vi "DB Message Loop.vi"(8 "error in (no error)":errorcluster, 11 "Message Queues":T1) -> (0 "error out":errorcluster)   [LabVIEW 2026, in "Database.lvlib"]
uses:
  Database.lvlib
  support/Architecture/Message Queue/All Message Queues.ctl
  support/Architecture/Message Queue/Message Cluster.ctl
  <vilib>/addons/database/Connection.llb/Conn ObjectReference.ctl
  controls/Loop Memory/DB Session Data.ctl
  controls/UI/Folder Name.ctl
  controls/Messaging Payloads/DB Query Request Payload.ctl
  controls/UI/UI List Type.ctl
  controls/UI/Data Entity.ctl
  controls/UI/Measurement Role Selection.ctl
  controls/Messaging Payloads/Fetch SensorID Payload.ctl
  controls/Messaging Payloads/MSG FetchSensorID Payload.ctl
  controls/Messaging Payloads/Fetch Config Payload.ctl
  controls/Messaging Payloads/MSG FetchConfiguration Payload.ctl
  Acquisition/Instrument Specifications Cluster Configuration.ctl
  controls/UI/Measurement Role.ctl
  controls/Messaging Payloads/Sensor FetchResponse.ctl
  controls/Messaging Payloads/Sensor CoreData Cluster.ctl
  controls/UI/Units Enum.ctl
  controls/UI/Signal Enum.ctl
  controls/UI/Settings Cluster.ctl
  controls/UI/Acq Settings.ctl
  Acquisition/Instrument Specifications Configuration.ctl
  controls/UI/Config Settings.ctl
  Processing/Processing Settings.ctl
  controls/Messaging Payloads/Sensor CoreData.ctl
  Processing/Test Parameters.ctl
  Processing/Test Parameters Cluster.ctl
  controls/UI/Test Sequence Context.ctl
  controls/UI/Direction.ctl
  controls/UI/Session Identfiers.ctl
  controls/UI/Test Sequence Settings.ctl
  controls/UI/Test Sequence State.ctl
  controls/UI/Test Sequence Enum.ctl
  controls/Controller/Stimulus Settings.ctl
  controls/Controller/Stimulus Outputs.ctl
  controls/Controller/Stimulus Output.ctl
  controls/Controller/Controller Core Data.ctl
  controls/Controller/Stimulus Output Configuration.ctl
  controls/Controller/Stimulus Role.ctl
  controls/Messaging Payloads/TestRuns Table Insert.ctl
  controls/Messaging Payloads/DB TestRunChannel Record.ctl
  controls/Messaging Payloads/Sensor InsertRequest.ctl
  controls/Diagnostics/Error Cluster.ctl
  controls/Messaging Payloads/Sensor Table Insert.ctl
  controls/Diagnostics/Error Payload.ctl
  controls/Messaging Payloads/Channel InsertRequest.ctl
  controls/Messaging Payloads/Channel CoreData Cluster.ctl
  controls/Messaging Payloads/Operator InsertRequest.ctl
  controls/Messaging Payloads/Processed Calibration Points.ctl
  controls/Messaging Payloads/Processed Calibration Point.ctl
  Processing/Test Status.ctl
  controls/Messaging Payloads/Calibration Point Table Insert.ctl
  controls/Diagnostics/Error_Payload.ctl
  <vilib>/addons/database/Connection.llb/DB Tools Open Connec (String).vi
  <vilib>/addons/database/Connection.llb/Conn Execute.vi
  <vilib>/addons/database/Recordset.llb/Rec Destroy - Connection.vi
  <vilib>/addons/database/Recordset.llb/Rec Fetch Integer Data (R).vi
  <vilib>/Utility/error.llb/Error Cluster From Error Code.vi
  <vilib>/ErrorRing/Error Ring.xnode
  <vilib>/addons/database/NI_Database_API.lvlib
  support/Architecture/Message Queue/Message Queue.lvlib
  Acquisition/Acquisition.lvlib
  Settings/Settings.lvlib
  Processing/Processing_Engine.lvlib
  Analysis/Analysis.lvlib
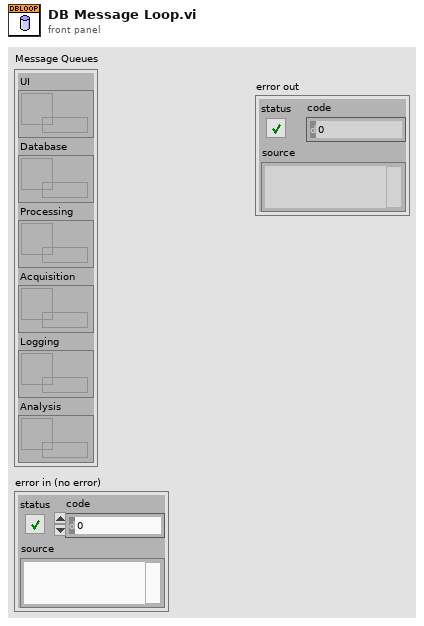
[diagram p1: front panel]
types:
  T1 = typedef "Message Queue.lvlib/All Message Queues.ctl" = cluster{"UI":refnum<queue>, "Database":refnum<queue>, "Processing":refnum<queue>, "Acquisition":refnum<queue>, "Logging":refnum<queue>, "Analysis":refnum<queue>}
  T2 = typedef "Folder Name.ctl" = enum16{"Data", "TDMS"}
  T3 = typedef "Settings.lvlib/Measurement Role Selection.ctl" = enum16{"Controller", "Reference", "UUT", "All"}
  T4 = typedef "UI List Type.ctl" = enum16{"Model Numbers", "Serial Numbers", "Operators", "Calibration Points", "Start Run Times"}
  T5 = typedef "Settings.lvlib/Measurement Role.ctl" = enum16{"Reference", "UUT"}
  T6 = typedef "DB Session Data.ctl" = cluster{"SensorID":i32[], "OperatorID":i32, "TestRunID":i32, "ChannelRecordIDs":i32[], "CalibrationSessionID":i32}
  T7 = typedef "NI_Database_API.lvlib/Conn ObjectReference.ctl" = refnum<k1>
  T8 = typedef "NI_Database_API.lvlib/Rec ObjectReference.ctl" = refnum<k1>
  T9 = typedef "DB Query Request Payload.ctl" = cluster{"1D Notifier":refnum<notifier>, "UI List Type":T4, "UI Device Type":T10, "Identifier":i32, "2D Notifier":refnum<notifier>, "Measurement Role Selection":T3}
  T10 = typedef "Settings.lvlib/Data Entity.ctl" = enum16{"Measurement", "Controller", " Test Configuration"}
  T11 = typedef "Database.lvlib/MSG FetchSensorID Payload.ctl" = cluster{"SensorID":i32, "Serial Number":string, "Model Number":string}
  T12 = typedef "Database.lvlib/Fetch SensorID Payload.ctl" = cluster{"Notifier":refnum<notifier>, "MSG FetchSensorID Payload":T11}
  T13 = typedef "MSG FetchConfiguration Payload.ctl" = cluster{"Serial Numbers":string[], "Hardware Settings Cluster":T14}
  T14 = typedef "Acquisition.lvlib/Instrument Specifications Cluster Configuration.ctl" = cluster{"Sensor ID *":i32, "Target Sample Rate (Hz) *":dbl, "Steady-State Duration (s) *":i32, "Allowed Tolerance (%) FS *":dbl, "Max Settling Timeout (s) *":i32, "Physical Channel":string, "Measurement Role":T5}
  T15 = typedef "Fetch Config Payload.ctl" = cluster{"Model Number":string, "Notifier":refnum<notifier>, "UI Device Type":T10}
  T16 = typedef "Sensor FetchResponse.ctl" = cluster{"Notifier":refnum<notifier>, "Sensor ID":i32}
  T17 = typedef "Settings.lvlib/Sensor CoreData Cluster.ctl" = cluster{"SerialNumber":string, "ModelNumber":string, "Min":dbl, "Max":dbl, "Units":T18, "Output Signal":T19, "SensorID":i32}
  T18 = typedef "Units Enum.ctl" = enum16{"PSI", "Deg C", "kPa", "GPM"}
  T19 = typedef "Signal Enum.ctl" = enum16{"4-20mA", "0-10V", "Thermocouple Type K"}
  T20 = typedef "Settings Cluster.ctl" = cluster{"Acq Settings":T21, "Processing Settings":T24, "Session Identifiers":T30, "Test Sequence Settings":T31, "Stimulus Settings":T34}
  T21 = typedef "Acq Settings.ctl" = cluster{"Instrument Specifications":T22, "Config Settings":T23}
  T22 = typedef "Acquisition.lvlib/Instrument Specifications Configuration.ctl" = T14[]
  T23 = typedef "Config Settings.ctl" = cluster{"Simulated Sensor Injection":dbl, "Base Device Name":string, "Simulation Mode":string}
  T24 = typedef "Processing_Engine.lvlib/Processing Settings.ctl" = cluster{"Sensor CoreData":T25, "Test Parameters":T26, "Measurement Roles":T5[], "Test Sequence Context":T28}
  T25 = typedef "Sensor CoreData.ctl" = T17[]
  T26 = typedef "Processing_Engine.lvlib/Test Parameters.ctl" = T27[]
  T27 = typedef "Settings.lvlib/Test Parameters Cluster.ctl" = cluster{"Steady-State Duration (s)":i32, "Allowed Tolerance (%) FS":dbl, "Max Settling Timeout (s)":i32}
  T28 = typedef "Settings.lvlib/Test Sequence Context.ctl" = cluster{"Direction":T29, "Cycle Number":i32, "Setpoint":dbl}
  T29 = typedef "Settings.lvlib/Direction.ctl" = enum16{"Acsending", "Descending"}
  T30 = typedef "Session Identfiers.ctl" = cluster{"SerialNumber":string[], "OperatorName":string}
  T31 = typedef "Test Sequence Settings.ctl" = cluster{"Test Sequence State":T32}
  T32 = typedef "Settings.lvlib/Test Sequence State.ctl" = cluster{"Test Sequence Enum":T33, "Point Index":i32, "Current Target":dbl, "Previous Target":dbl, "Simulation?":bool, "Direction":T29, "Transition Active?":bool, "Cycle Number":i32}
  T33 = typedef "Test Sequence Enum.ctl" = enum16{"Idle", "Start Point", "Point Complete", "Test Complete", "Abort Test", "Reset"}
  T34 = typedef "Settings.lvlib/Stimulus Settings.ctl" = cluster{"Stimulus Outputs":T35}
  T35 = typedef "Settings.lvlib/Stimulus Outputs.ctl" = T36[]
  T36 = typedef "Settings.lvlib/Stimulus Output.ctl" = cluster{"Controller Core Data":T37, "Stimulus Output Configuration":T38}
  T37 = typedef "Settings.lvlib/Controller Core Data.ctl" = cluster{"Min":dbl, "Max":dbl, "Units":T18, "Input Signal Type":T19, "Input Signal Min":dbl, "Input Signal Max":dbl}
  T38 = typedef "Settings.lvlib/Stimulus Output Configuration.ctl" = cluster{"DAQmx AO Physical Channel":tag, "Role":T39, "Model Numbers":string, "Serial Numbers":string, "Row":i32}
  T39 = typedef "Stimulus Role.ctl" = enum16{"Pressure Controller", "Temperature Controller"}
  T40 = typedef "TestRuns Table Insert.ctl" = cluster{"RunStartTime":string, "OperatorID":i32, "TestResult":string, "CalibrationSessionID":i32}
  T41 = typedef "Database.lvlib/DB TestRunChannel Record.ctl" = cluster{"TestRunID":i32, "SensorID":i32, "HardwareRow":i32, "PhysicalChannel":string, "FinalStatus":string, "MeasurementRole":string}
  T42 = typedef "Settings.lvlib/Sensor Table Insert.ctl" = cluster{"SerialNumber":string, "ModelNumber":string, "Min":dbl, "Max":dbl, "Units":T18, "Output Signal":T19}
  T43 = typedef "Sensor InsertRequest.ctl" = cluster{"Notifier":refnum<notifier>, "Sensor CoreData":T17}
  T44 = typedef "Error Cluster.ctl" = errorcluster
  T45 = typedef "Error Payload.ctl" = cluster{"Error Cluster":T44, "Message":string}
  T46 = typedef "Settings.lvlib/Channel CoreData Cluster.ctl" = cluster{"RunID":i32, "SensorID":i32, "HardwareRow":i32, "PhysicalChannel":string}
  T47 = typedef "Settings.lvlib/Channel InsertRequest.ctl" = cluster{"Notifier":refnum<notifier>, "Channel CoreData":T46}
  T48 = typedef "Operator InsertRequest.ctl" = cluster{"Notifier":refnum<notifier>, "OperatorName":string, "BadgeNumber":string, "IsActive":i32}
  T49 = typedef "Processed Calibration Points.ctl" = T50[]
  T50 = typedef "Processed Calibration Point.ctl" = cluster{"Reference Value":dbl, "Measured Value":dbl, "AccuracyPercentFS":dbl, "Pass/Fail":bool, "Setpoint":dbl, "Cycle Number":i32, "Direction":T29, "Test Status":T51}
  T51 = typedef "Analysis.lvlib/Test Status.ctl" = enum16{"Overall Pass", "Overall Fail", "Test Running"}
  T52 = typedef "Calibration Point Table Insert.ctl" = cluster{"TestRunID":i32, "ChannelRecordID":i32, "Setpoint":dbl, "MeasuredValue":dbl, "AccuracyPercentFS":dbl, "PassFail":bool, "ReferenceValue":dbl, "Cycle Number":i32, "Direction":string, "SensorID":i32}
  T53 = typedef "Error_Payload.ctl" = cluster{"status":bool, "error_code":i32, "description":string, "source_loop":string}
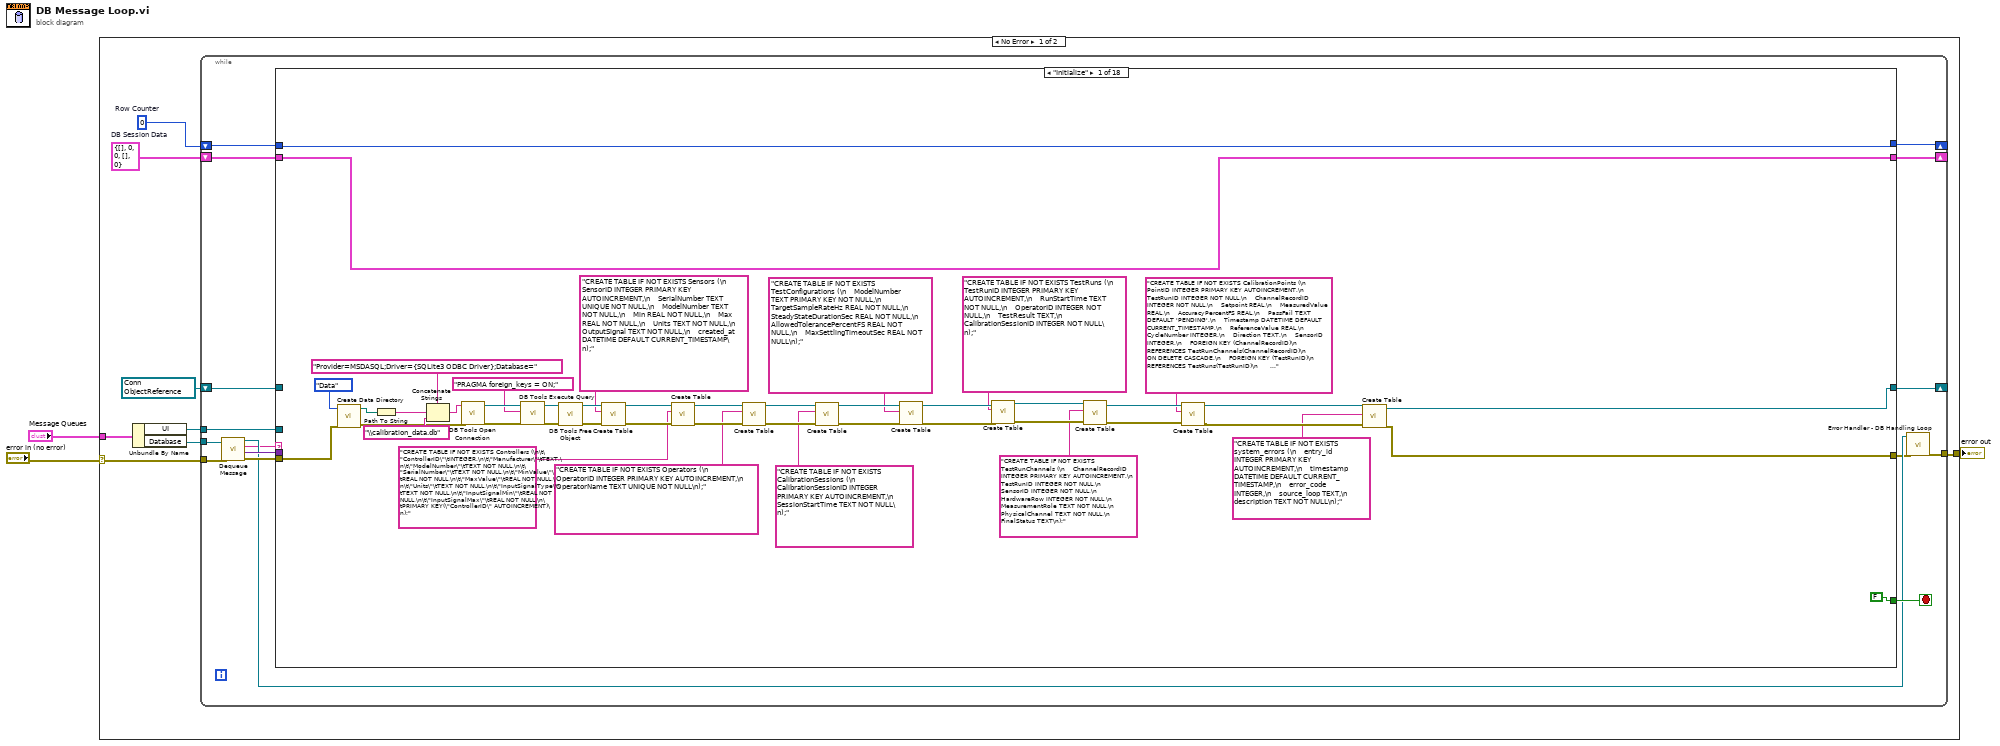
[diagram p0: block diagram]
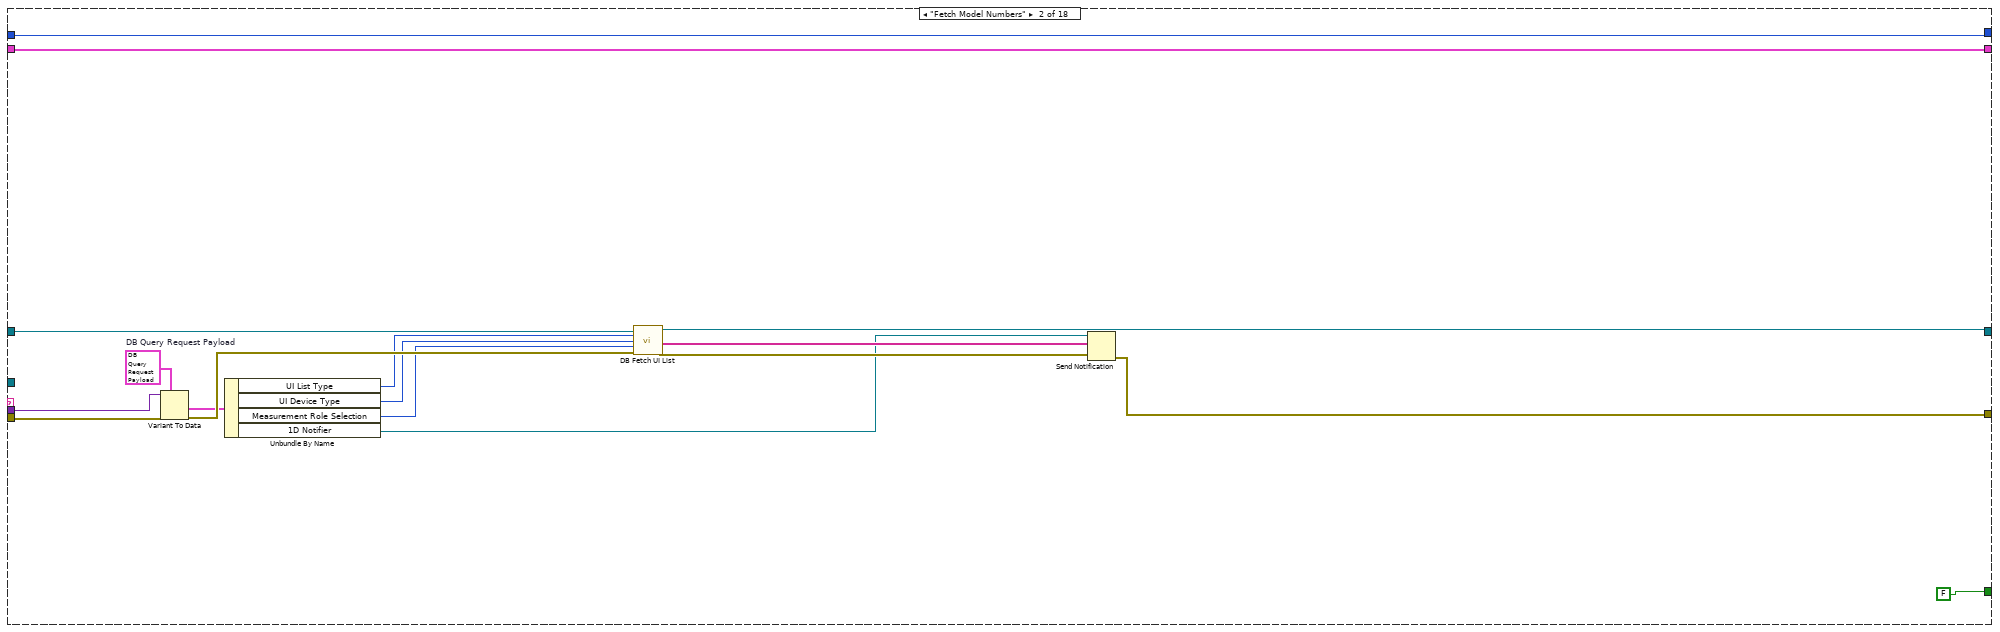
[diagram p2: hidden frame]
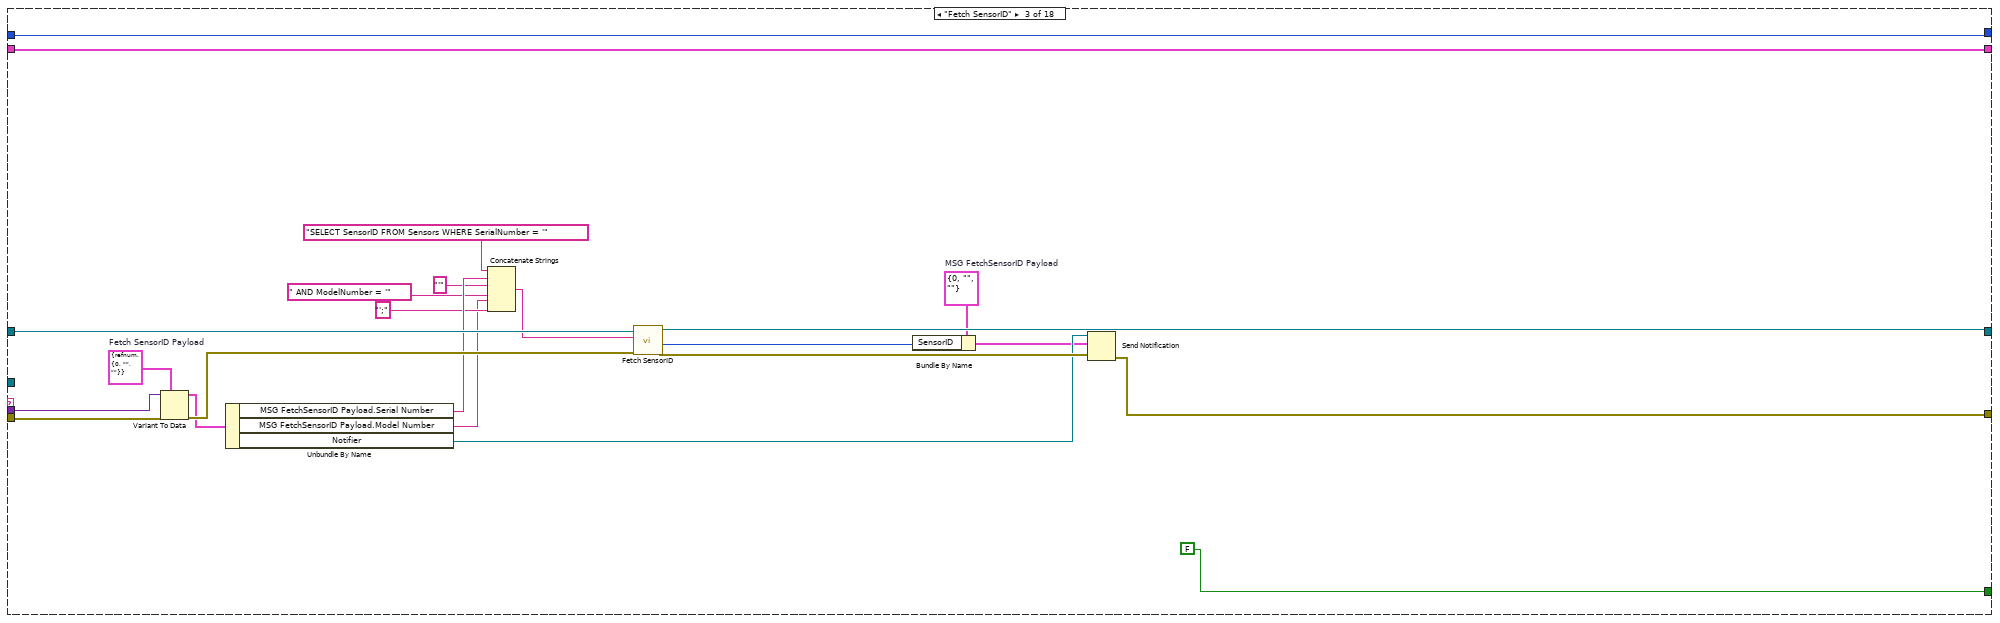
[diagram p3: hidden frame]
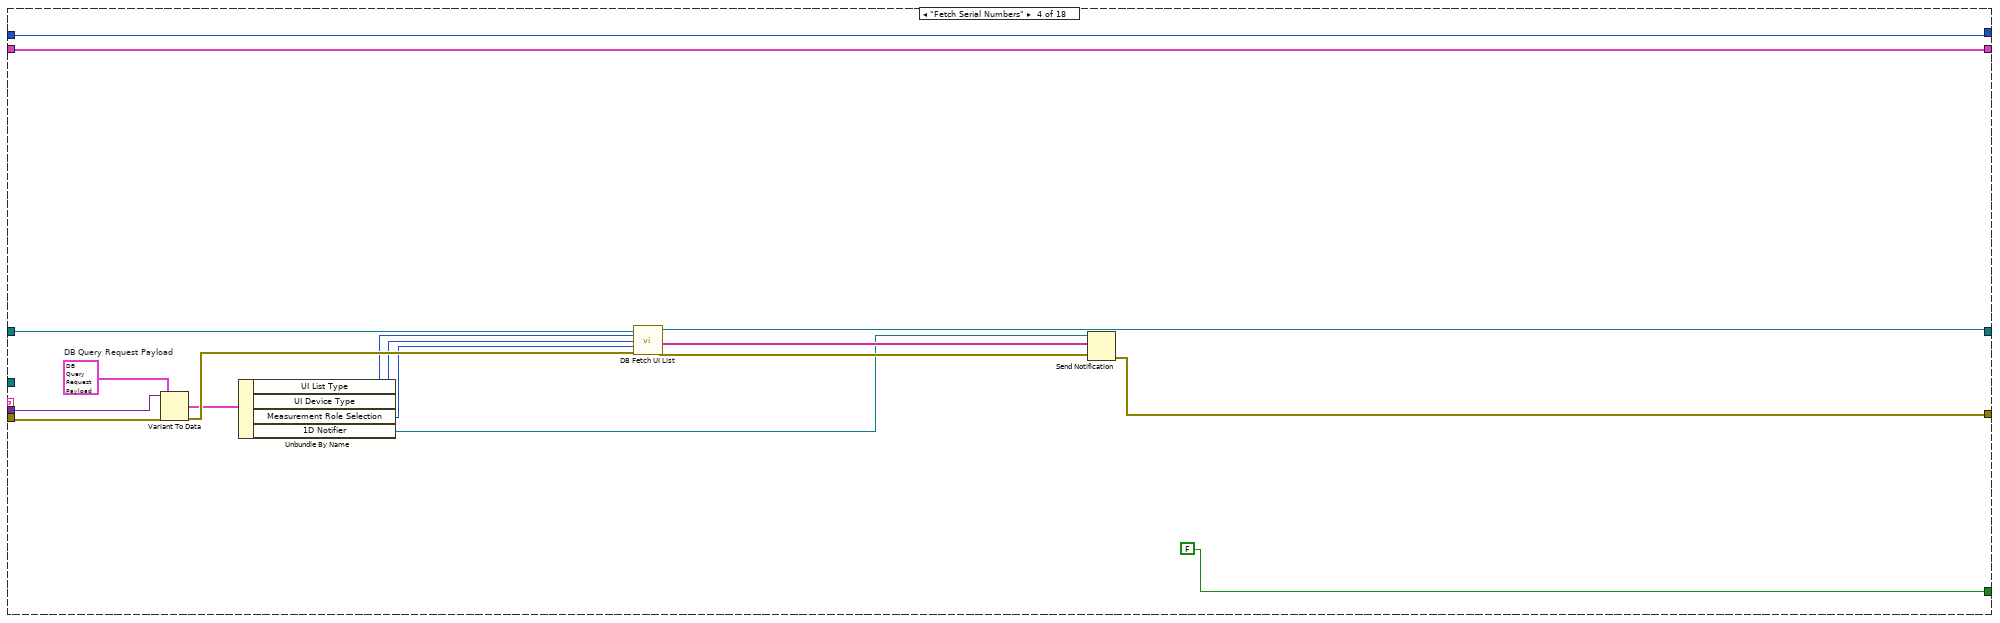
[diagram p4: hidden frame]
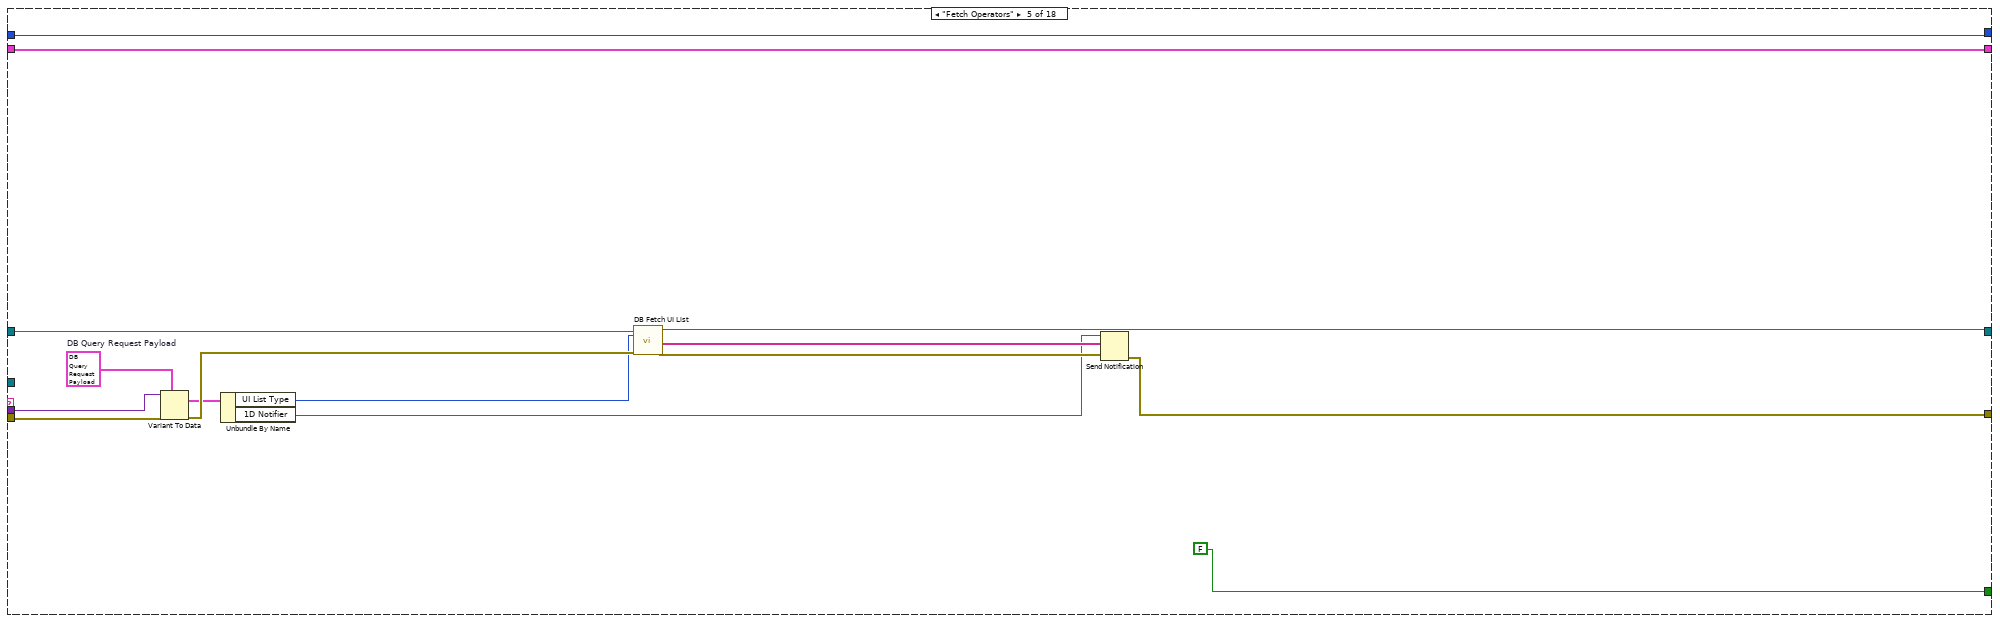
[diagram p5: hidden frame]
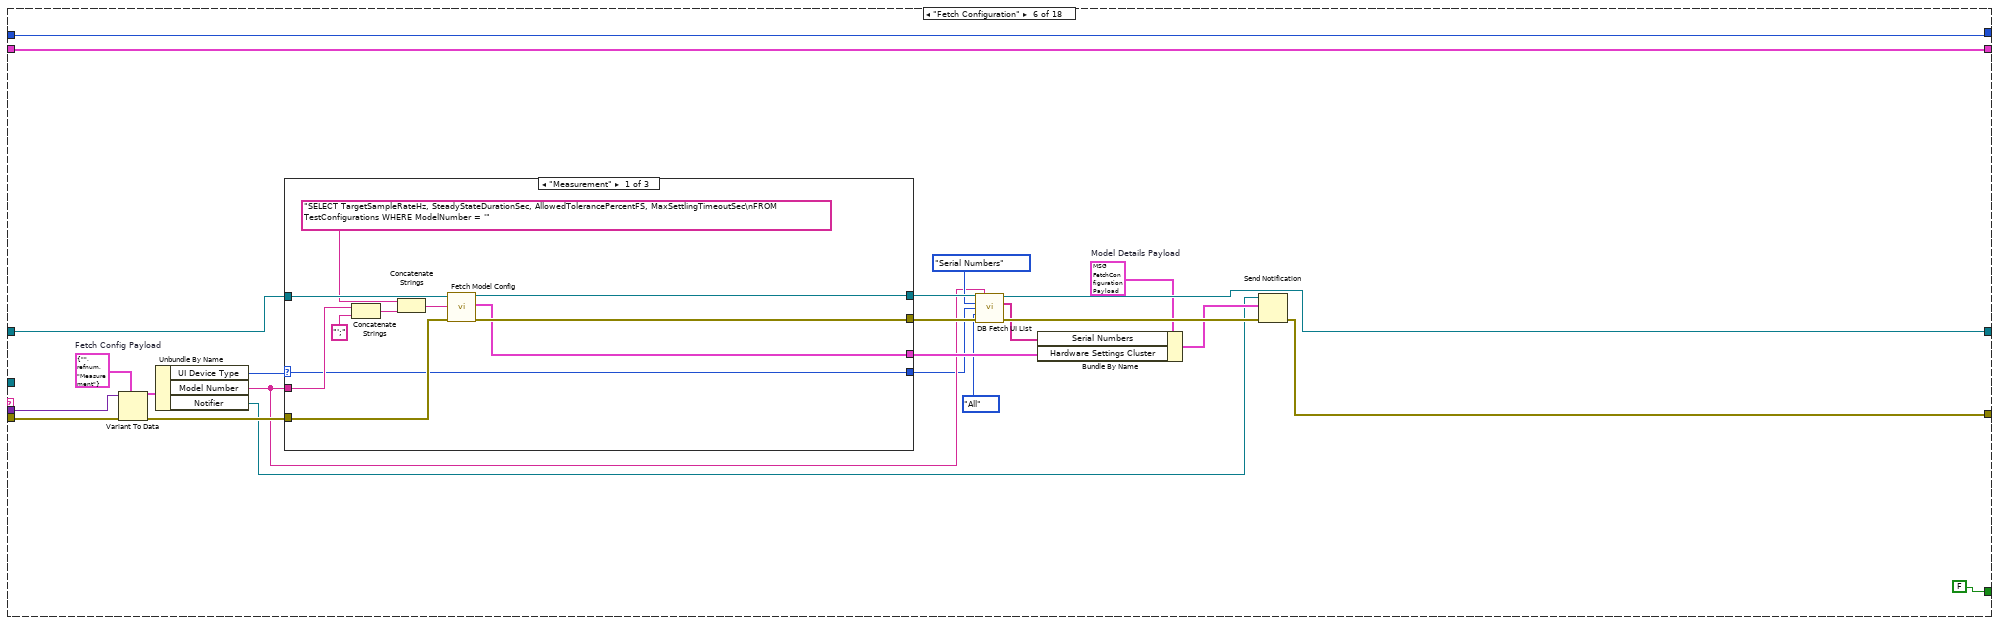
[diagram p6: hidden frame]
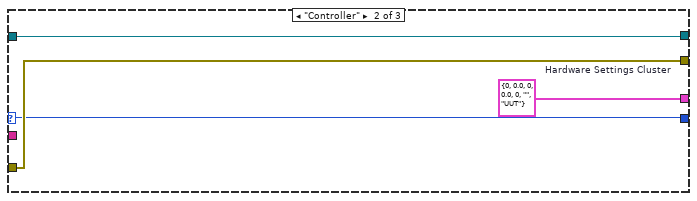
[diagram p7: hidden frame]
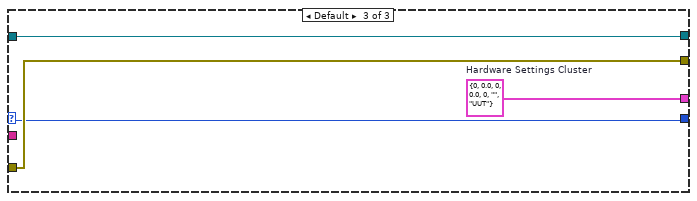
[diagram p8: hidden frame]
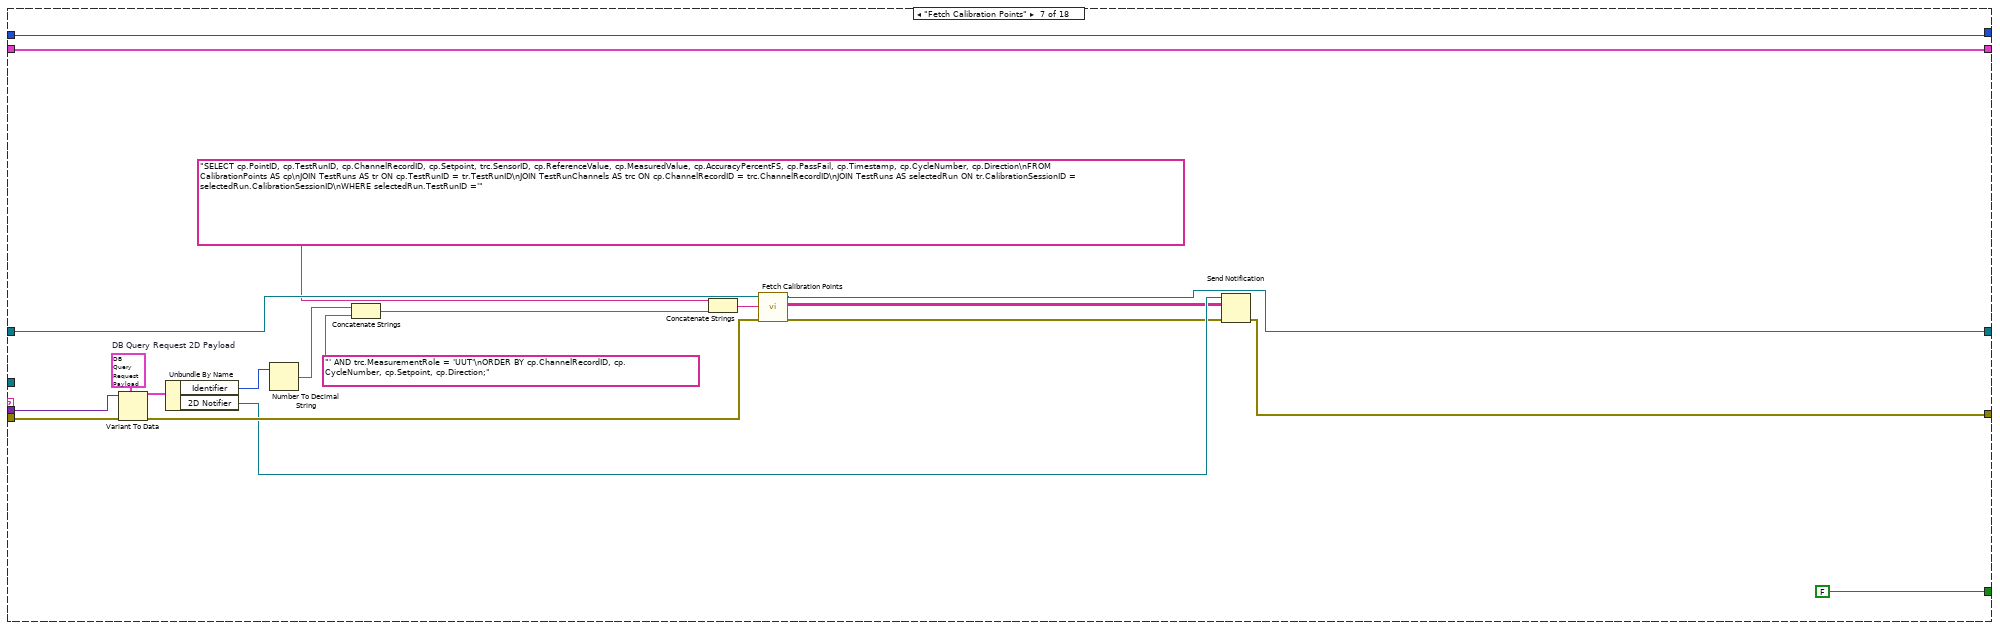
[diagram p9: hidden frame]
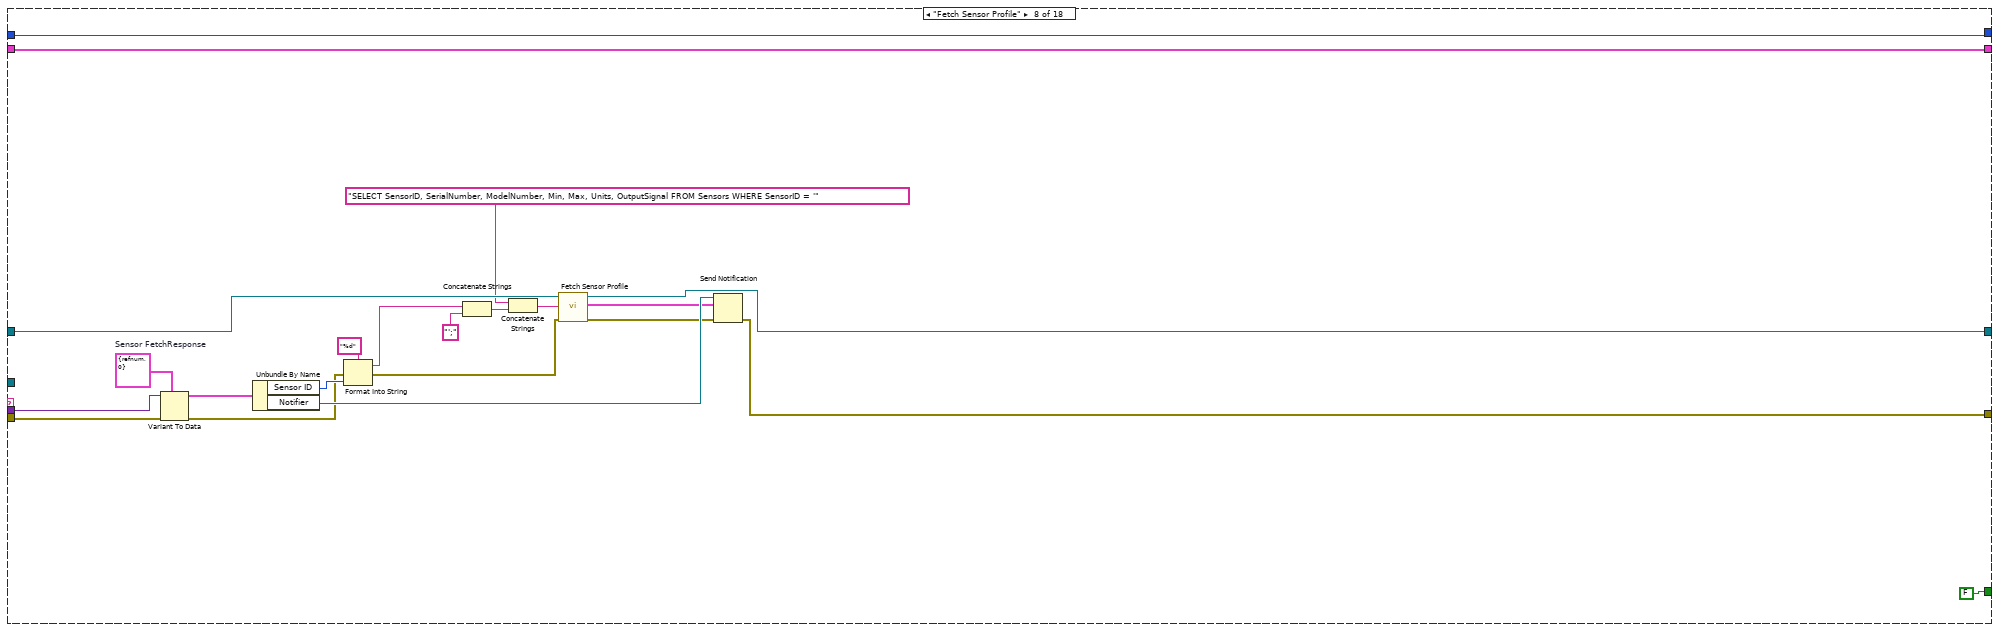
[diagram p10: hidden frame]
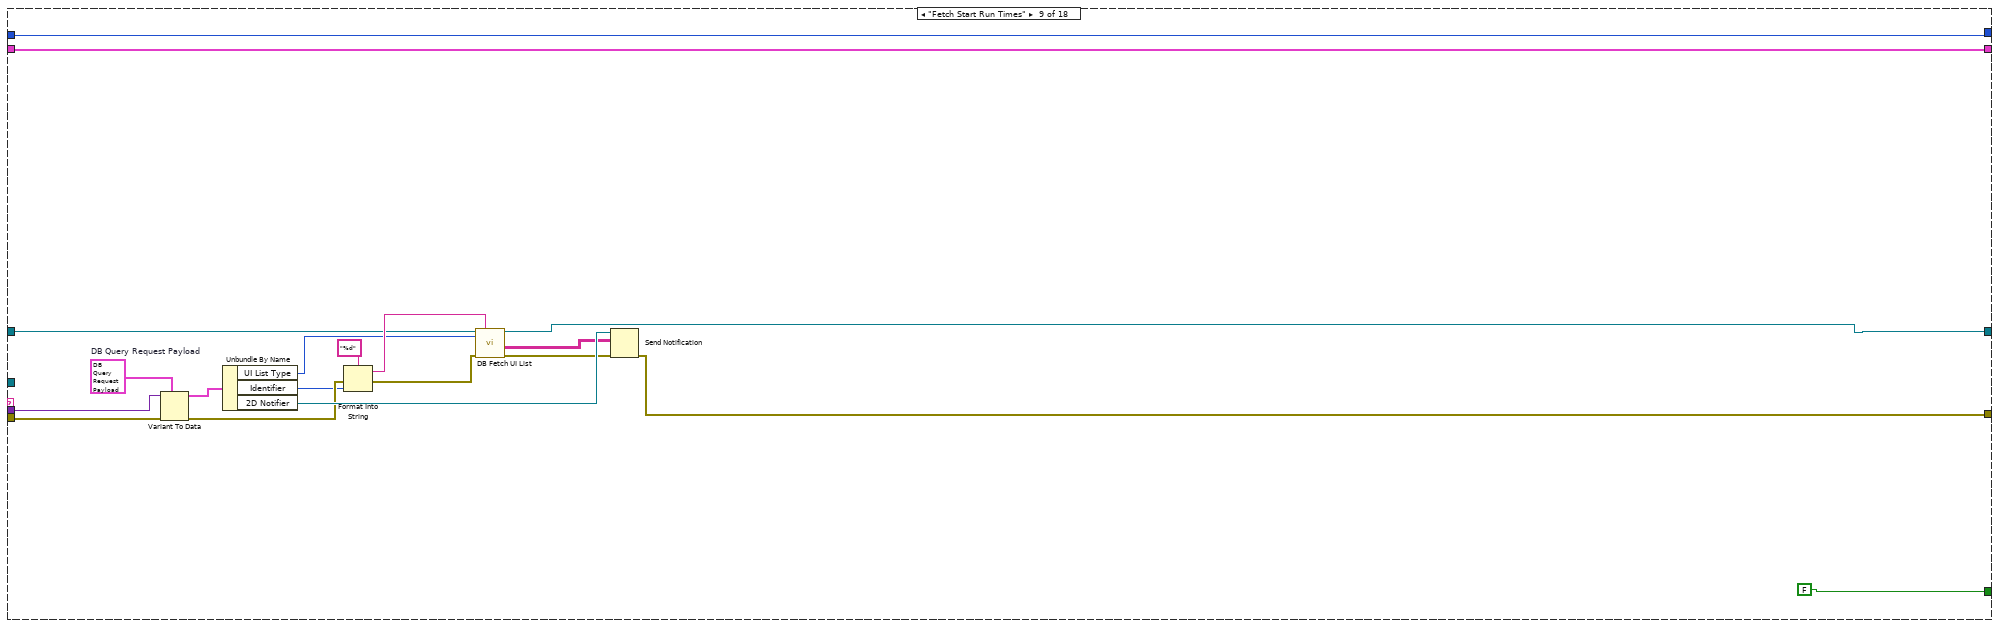
[diagram p11: hidden frame]
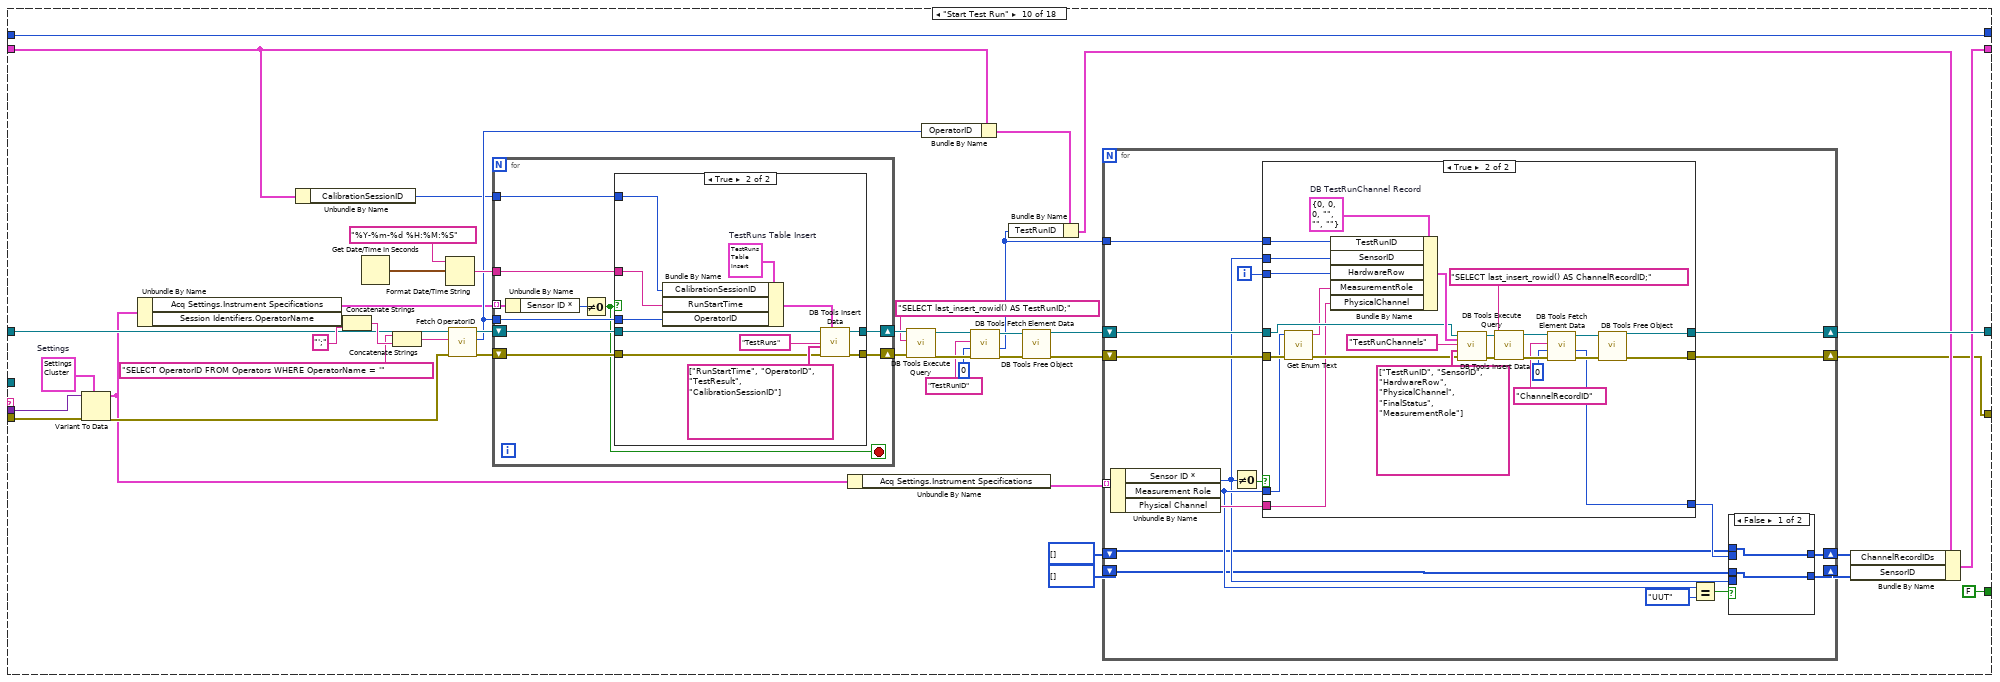
[diagram p12: hidden frame]
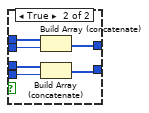
[diagram p13: hidden frame]
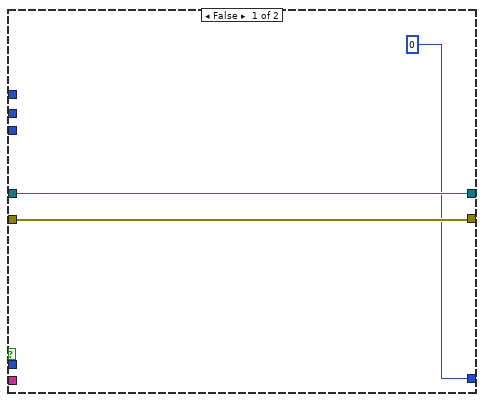
[diagram p14: hidden frame]
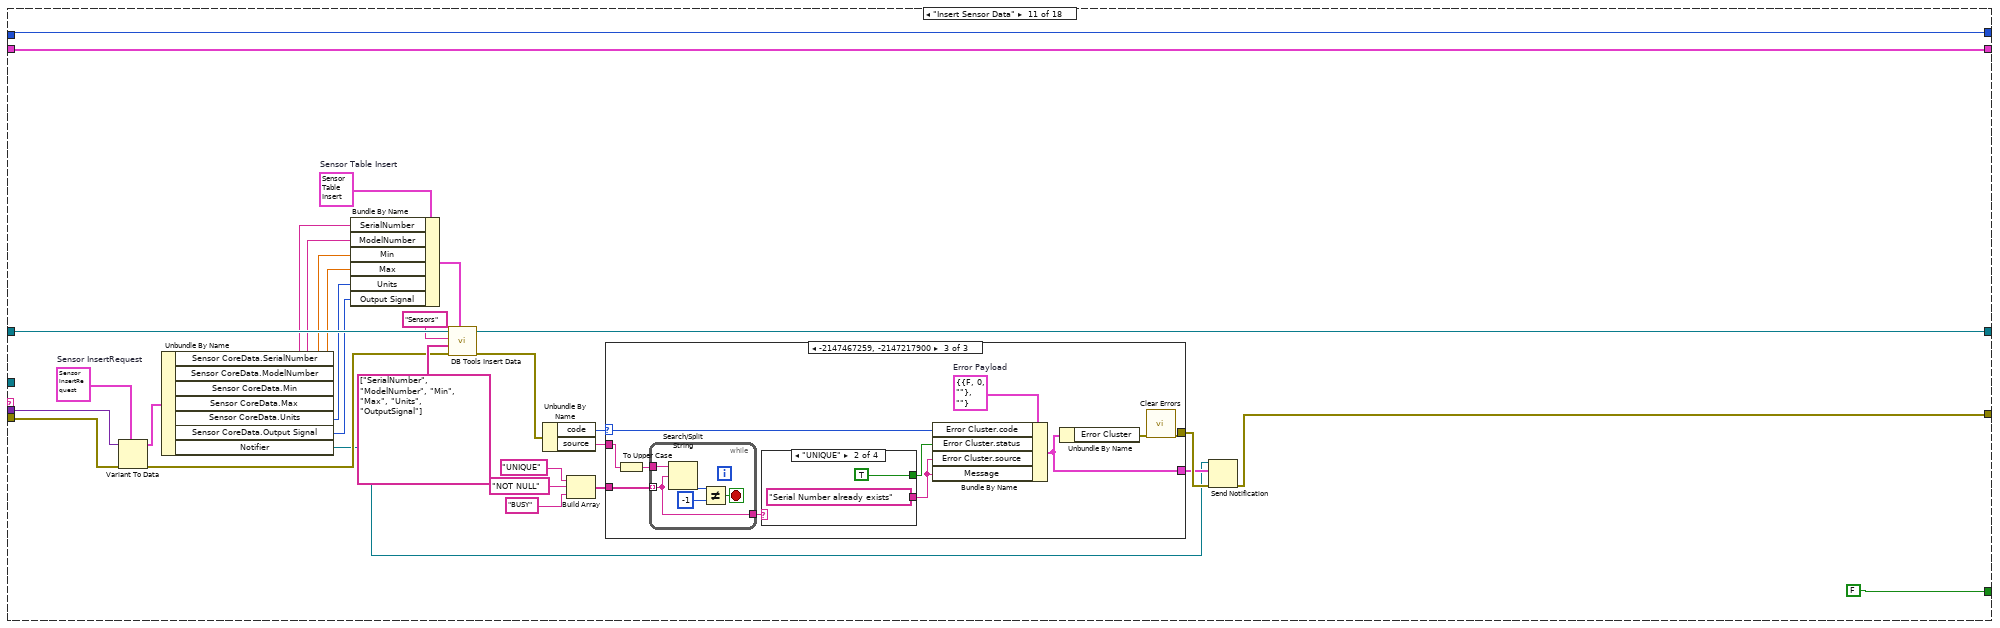
[diagram p16: hidden frame]
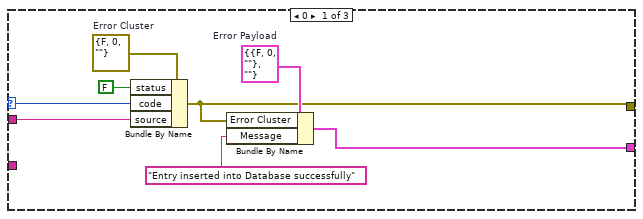
[diagram p17: hidden frame]
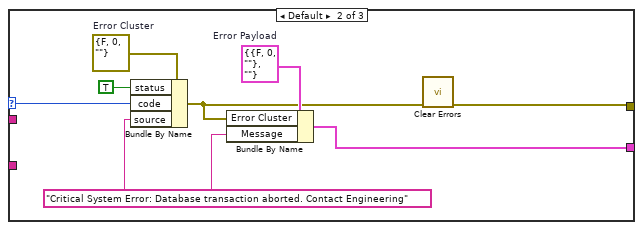
[diagram p18: hidden frame]
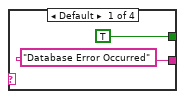
[diagram p19: hidden frame]
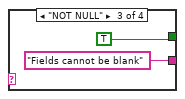
[diagram p20: hidden frame]
diagram:
  n1 = case shown="No Error" "error in (no error)" {
    selector: "error in (no error)" -> [w9 w748]
    tunnel: [w10 w748] -> w3
    tunnel: "Message Queues" -> [w8 _]
    frame No Error {
      w5 = T6 {"SensorID"=[], "OperatorID"=0, "TestRunID"=0, "ChannelRecordIDs"=[], "CalibrationSessionID"=0}  # DB Session Data
      w11 = T7 refnum items=["Connection"] ("connection reference")
      w4 = 0  # Row Counter
      n2 = Unbundle By Name(w8) -> ("UI"=w6:refnum<queue>, "Database"=w7:refnum<queue>)
      n3 = while {
        tunnel: w9 -> [w27]
        tunnel: [w24] -> w10
        shift-right: [w22] -> _
        shift-left: w11 -> [w21]
        shift-right: [w19] -> _
        shift-left: w4 -> [w20]
        tunnel: w7 -> [w18]
        tunnel: w6 -> [w16]
        shift-right: [w14] -> _
        shift-left: w5 -> [w13]
        stop <- w25 stop-if-true
        n4 = call "Dequeue Message.vi"("error in (no error)"=w27, "Message Queue"=w18) -> ("error out"=w26:errorcluster, "Message Data"=w23:variant, "Message"=w15:string, "dup Message Queue"=w17:refnum<queue>)  [unwired: 6 in]
        n5 = case shown="\"Initialize\"" w15 {
          selector: w15 -> [_ _ _ _ _ _ _ _ _ _ _ _ _ _ _ _ _ w739]
          tunnel: w26 -> [w66 w88 w111 w128 w143 w167 w206 w228 w247 w269 w399 w468 w532 w575 w614 w695 w717 _]
          tunnel: [FALSE FALSE FALSE FALSE FALSE FALSE FALSE FALSE FALSE FALSE FALSE FALSE FALSE FALSE FALSE FALSE TRUE FALSE] -> w25
          tunnel: [w37 w83 w106 w123 w137 w159 w201 w220 w243 w255 w386 w456 w520 w580 w600 w682 w725 w738] -> w12
          tunnel: w23 -> [_ w78 w101 w117 w142 w151 w199 w213 w241 w290 w398 w467 w510 _ w597 w694 _ _]
          tunnel: [w36 w82 w105 w122 w136 w157 w192 w215 w234 w262 w379 w449 w511 w579 w610 w684 _ w737] -> w22
          tunnel: w21 -> [_ w85 w108 w125 w139 w164 w203 w225 w237 w266 w394 w464 w529 w592 w612 w688 w721 w737]
          tunnel: w20 -> [w71 w87 w110 w127 w141 w166 w205 w227 w246 w291 w397 w441 w531 w593 w613 w689 w723 w736]
          tunnel: [w71 w87 w110 w127 w141 w166 w205 w227 w246 w291 w397 w441 w531 w593 w613 w690 w723 w736] -> w19
          tunnel: w16 -> [_ _ _ _ _ _ _ _ _ _ _ _ _ _ _ _ _ _]
          tunnel: [w62 w79 w102 w118 w130 w154 w200 w218 w242 w256 w381 w451 w513 w576 w599 w677 w718 w735] -> w14
          tunnel: w13 -> [w62 w79 w102 w118 w130 w154 w200 w218 w242 w254 w381 w451 w513 w578 w599 w677 w718 w735]
          frame "Initialize" {
            n6 = call "Create Data Directory.vi"("error in (no error)"=w66, "Folder Name"=Folder_Name."Data") -> ("error out"=w65:errorcluster, "file path"=w64:path)  [unwired: 8 in]
            n7 = Path To String(path=w64) -> (string=w70:string)
            n8 = Concatenate Strings("Provider=MSDASQL;Driver={SQLite3 ODBC Driver};Database=", w70, "\\calibration_data.db" ("string")) -> (w67:string)
            n9 = call-poly <vilib>:"DB Tools Open Connection.vi"("error in (no error)"=w65, "connection information"=w67) -> ("error out"=w58:errorcluster, "connection reference"=w59:T7)  [unwired: 6 in]
            n10 = call-poly <vilib>:"DB Tools Execute Query.vi"("error in (no error)"=w58, "SQL query"="PRAGMA foreign_keys = ON;", "connection reference"=w59) -> ("error out"=w61:errorcluster, "recordset reference"=w60:T8)  [unwired: 5 in]
            n11 = call-poly <vilib>:"DB Tools Free Object.vi"("error in (no error)"=w61, "recordset reference"=w60) -> ("error out"=w56:errorcluster, "connection reference"=w54:T7)  [unwired: 8 in]
            n12 = call "Create Table.vi"("error in (no error)"=w56, "SQL Statement"="CREATE TABLE IF NOT EXISTS Sensors (\n    SensorID INTEGER PRIMARY KEY AUTOINCREMENT,\n    SerialNumber TEXT UNIQUE NOT NULL,\n    ModelNumber TEXT NOT NULL,\n    Min REAL NOT NULL,\n    Max REAL NOT NULL,\n    Units TEXT NOT NULL,\n    OutputSignal TEXT NOT NULL,\n    created_at DATETIME DEFAULT CURRENT_TIMESTAMP\n);", "Refnum in"=w54) -> ("error out"=w55:errorcluster, "Refnum out"=w53:T7)  [unwired: 7 in]
            n13 = call "Create Table.vi"("error in (no error)"=w55, "SQL Statement"="CREATE TABLE IF NOT EXISTS Controllers (\n\t\"ControllerID\"\tINTEGER,\n\t\"Manufacturer\"\tTEXT,\n\t\"ModelNumber\"\tTEXT NOT NULL,\n\t\"SerialNumber\"\tTEXT NOT NULL,\n\t\"MinValue\"\tREAL NOT NULL,\n\t\"MaxValue\"\tREAL NOT NULL,\n\t\"Units\"\tTEXT NOT NULL,\n\t\"InputSignalType\"\tTEXT NOT NULL,\n\t\"InputSignalMin\"\tREAL NOT NULL,\n\t\"InputSignalMax\"\tREAL NOT NULL,\n\tPRIMARY KEY(\"ControllerID\" AUTOINCREMENT)\n);" ("SQL query"), "Refnum in"=w53) -> ("error out"=w52:errorcluster, "Refnum out"=w51:T7)  [unwired: 7 in]
            n14 = call "Create Table.vi"("error in (no error)"=w52, "SQL Statement"="CREATE TABLE IF NOT EXISTS Operators (\n    OperatorID INTEGER PRIMARY KEY AUTOINCREMENT,\n    OperatorName TEXT UNIQUE NOT NULL\n);", "Refnum in"=w51) -> ("error out"=w49:errorcluster, "Refnum out"=w50:T7)  [unwired: 7 in]
            n15 = call "Create Table.vi"("error in (no error)"=w49, "SQL Statement"="CREATE TABLE IF NOT EXISTS CalibrationSessions (\n    CalibrationSessionID INTEGER PRIMARY KEY AUTOINCREMENT,\n    SessionStartTime TEXT NOT NULL\n);" ("SQL query"), "Refnum in"=w50) -> ("error out"=w48:errorcluster, "Refnum out"=w47:T7)  [unwired: 7 in]
            n16 = call "Create Table.vi"("error in (no error)"=w48, "SQL Statement"="CREATE TABLE IF NOT EXISTS TestConfigurations (\n    ModelNumber TEXT PRIMARY KEY NOT NULL,\n    TargetSampleRateHz REAL NOT NULL,\n    SteadyStateDurationSec REAL NOT NULL,\n    AllowedTolerancePercentFS REAL NOT NULL,\n    MaxSettlingTimeoutSec REAL NOT NULL\n);", "Refnum in"=w47) -> ("error out"=w46:errorcluster, "Refnum out"=w45:T7)  [unwired: 7 in]
            n17 = call "Create Table.vi"("error in (no error)"=w46, "SQL Statement"="CREATE TABLE IF NOT EXISTS TestRuns (\n    TestRunID INTEGER PRIMARY KEY AUTOINCREMENT,\n    RunStartTime TEXT NOT NULL,\n    OperatorID INTEGER NOT NULL,\n    TestResult TEXT,\n    CalibrationSessionID INTEGER NOT NULL\n);", "Refnum in"=w45) -> ("error out"=w44:errorcluster, "Refnum out"=w43:T7)  [unwired: 7 in]
            n18 = call "Create Table.vi"("error in (no error)"=w44, "SQL Statement"="CREATE TABLE IF NOT EXISTS TestRunChannels (\n    ChannelRecordID INTEGER PRIMARY KEY AUTOINCREMENT,\n    TestRunID INTEGER NOT NULL,\n    SensorID INTEGER NOT NULL,\n    HardwareRow INTEGER NOT NULL,\n    MeasurementRole TEXT NOT NULL,\n    PhysicalChannel TEXT NOT NULL,\n    FinalStatus TEXT\n);" ("SQL query"), "Refnum in"=w43) -> ("error out"=w40:errorcluster, "Refnum out"=w41:T7)  [unwired: 7 in]
            n19 = call "Create Table.vi"("error in (no error)"=w40, "SQL Statement"="CREATE TABLE IF NOT EXISTS CalibrationPoints (\n    PointID INTEGER PRIMARY KEY AUTOINCREMENT,\n    TestRunID INTEGER NOT NULL,\n    ChannelRecordID INTEGER NOT NULL,\n    Setpoint REAL,\n    MeasuredValue REAL,\n    AccuracyPercentFS REAL,\n    PassFail TEXT DEFAULT 'PENDING',\n    Timestamp DATETIME DEFAULT CURRENT_TIMESTAMP,\n    ReferenceValue REAL,\n    CycleNumber INTEGER,\n    Direction TEXT,\n    SensorID INTEGER,\n    FOREIGN KEY (ChannelRecordID)\n        REFERENCES TestRunChannels(ChannelRecordID)\n        ON DELETE CASCADE,\n    FOREIGN KEY (TestRunID)\n        REFERENCES TestRuns(TestRunID)\n        ON DELETE CASCADE\n);", "Refnum in"=w41) -> ("error out"=w38:errorcluster, "Refnum out"=w39:T7)  [unwired: 7 in]
            n20 = call "Create Table.vi"("error in (no error)"=w38, "SQL Statement"="CREATE TABLE IF NOT EXISTS system_errors (\n    entry_id INTEGER PRIMARY KEY AUTOINCREMENT,\n    timestamp DATETIME DEFAULT CURRENT_TIMESTAMP,\n    error_code INTEGER,\n    source_loop TEXT,\n    description TEXT NOT NULL\n);" ("SQL query"), "Refnum in"=w39) -> ("error out"=w37:errorcluster, "Refnum out"=w36:T7)  [unwired: 7 in]
          }
          frame "Fetch Model Numbers" {
            w81 = T9 {"1D Notifier"=refnum, "UI List Type"=enum."Model Numbers", "UI Device Type"=enum."Measurement", "Identifier"=0, "2D Notifier"=refnum, "Measurement Role Selection"=enum."Controller"}  # DB Query Request Payload
            n21 = Variant To Data(error in=w88, type=w81, Variant=w78) -> (data=w80:T9, error out=w86:errorcluster)
            n22 = Unbundle By Name(w80) -> ("UI List Type"=w76:T4, "UI Device Type"=w75:T10, "Measurement Role Selection"=w73:T3, "1D Notifier"=w74:refnum<notifier>)
            n23 = call "DB Fetch UI List.vi"("Refnum in"=w85, "UI List Type"=w76, "UI Device Type"=w75, "Measurement Role"=w73, "error in (no error)"=w86) -> ("Refnum out"=w82:T7, "1D Results"=w77:string[], "error out"=w84:errorcluster)  [unwired: 7 in, 1 out]
            n24 = Send Notification(notification=w77, notifier=w74, error in (no error)=w84) -> (error out=w83:errorcluster)  [unwired: 1 out]
          }
          frame "Fetch SensorID" {
            w93 = T11 {"SensorID"=0, "Serial Number"="", "Model Number"=""}  # MSG FetchSensorID Payload
            w104 = T12 {"Notifier"=refnum, "MSG FetchSensorID Payload"={"SensorID"=0, "Serial Number"="", "Model Number"=""}}  # Fetch SensorID Payload
            n25 = Variant To Data(error in=w111, type=w104, Variant=w101) -> (data=w95:T12, error out=w109:errorcluster)
            n26 = Unbundle By Name(w95) -> ("MSG FetchSensorID Payload.Serial Number"=w99:string, "MSG FetchSensorID Payload.Model Number"=w90:string, "Notifier"=w103:refnum<notifier>)
            n27 = Concatenate Strings("SELECT SensorID FROM Sensors WHERE SerialNumber = '" ("SQL query"), w99, "'", " AND ModelNumber = '", w90, "';") -> (w96:string)
            n28 = call "Fetch SensorID.vi"("error in (no error)"=w109, "SQL query"=w96, "Refnum in"=w108) -> ("error out"=w107:errorcluster, "SensorID"=w94:i32, "Refnum out"=w105:T7)  [unwired: 6 in]
            n29 = Bundle By Name(cluster=w93, "SensorID"=w94) -> (w92:T11)
            n30 = Send Notification(notification=w92, notifier=w103, error in (no error)=w107) -> (error out=w106:errorcluster)  [unwired: 1 out]
          }
          frame "Fetch Serial Numbers" {
            w120 = T9 {"1D Notifier"=refnum, "UI List Type"=enum."Model Numbers", "UI Device Type"=enum."Measurement", "Identifier"=0, "2D Notifier"=refnum, "Measurement Role Selection"=enum."Controller"}  # DB Query Request Payload
            n31 = Variant To Data(error in=w128, type=w120, Variant=w117) -> (data=w119:T9, error out=w126:errorcluster)
            n32 = Unbundle By Name(w119) -> ("UI List Type"=w113:T4, "UI Device Type"=w114:T10, "Measurement Role Selection"=w115:T3, "1D Notifier"=w116:refnum<notifier>)
            n33 = call "DB Fetch UI List.vi"("Refnum in"=w125, "UI List Type"=w113, "UI Device Type"=w114, "Measurement Role"=w115, "error in (no error)"=w126) -> ("Refnum out"=w122:T7, "1D Results"=w121:string[], "error out"=w124:errorcluster)  [unwired: 7 in, 1 out]
            n34 = Send Notification(notification=w121, notifier=w116, error in (no error)=w124) -> (error out=w123:errorcluster)  [unwired: 1 out]
          }
          frame "Fetch Operators" {
            w134 = T9 {"1D Notifier"=refnum, "UI List Type"=enum."Model Numbers", "UI Device Type"=enum."Measurement", "Identifier"=0, "2D Notifier"=refnum, "Measurement Role Selection"=enum."Controller"}  # DB Query Request Payload
            n35 = Variant To Data(error in=w143, type=w134, Variant=w142) -> (data=w133:T9, error out=w140:errorcluster)
            n36 = Unbundle By Name(w133) -> ("UI List Type"=w132:T4, "1D Notifier"=w131:refnum<notifier>)
            n37 = call "DB Fetch UI List.vi"("Refnum in"=w139, "UI List Type"=w132, "error in (no error)"=w140) -> ("Refnum out"=w136:T7, "1D Results"=w135:string[], "error out"=w138:errorcluster)  [unwired: 9 in, 1 out]
            n38 = Send Notification(notification=w135, notifier=w131, error in (no error)=w138) -> (error out=w137:errorcluster)  [unwired: 1 out]
          }
          frame "Fetch Configuration" {
            w156 = T13 {"Serial Numbers"=[], "Hardware Settings Cluster"={"Sensor ID *"=0, "Target Sample Rate (Hz) *"=0.0, "Steady-State Duration (s) *"=0, "Allowed Tolerance (%) FS *"=0.0, "Max Settling Timeout (s) *"=5, "Physical Channel"="", "Measurement Role"=enum."Reference"}}  # Model Details Payload
            w163 = T15 {"Model Number"="", "Notifier"=refnum, "UI Device Type"=enum."Measurement"}  # Fetch Config Payload
            n39 = Variant To Data(error in=w167, type=w163, Variant=w151) -> (data=w162:T15, error out=w165:errorcluster)
            n40 = Unbundle By Name(w162) -> ("UI Device Type"=w149:T10, "Model Number"=w148:string, "Notifier"=w147:refnum<notifier>)
            n41 = case shown="\"Measurement\"" w149 {
              selector: w149 -> [w169 w180 w184]
              tunnel: w165 -> [w178 w182 w186]
              tunnel: w164 -> [w177 w183 w187]
              tunnel: [w176 w182 w186] -> w161
              tunnel: [w173 w183 w187] -> w158
              tunnel: [w172 w181 w185] -> w153
              tunnel: w148 -> [w170 _ _]
              tunnel: [w169 w180 w184] -> w146
              frame "Measurement" {
                n42 = Concatenate Strings(w170, "';") -> (w171:string)
                n43 = Concatenate Strings("SELECT TargetSampleRateHz, SteadyStateDurationSec, AllowedTolerancePercentFS, MaxSettlingTimeoutSec\nFROM TestConfigurations WHERE ModelNumber = '", w171) -> (w175:string)
                n44 = call "Fetch Model Config.vi"("error in (no error)"=w178, "SQL Query"=w175, "Refnum in"=w177) -> ("error out"=w176:errorcluster, "Hardware Settings Cluster"=w172:T14, "Refnum out"=w173:T7)  [unwired: 6 in]
              }
              frame "Controller" {
                w181 = T14 {"Sensor ID *"=0, "Target Sample Rate (Hz) *"=0.0, "Steady-State Duration (s) *"=0, "Allowed Tolerance (%) FS *"=0.0, "Max Settling Timeout (s) *"=0, "Physical Channel"="", "Measurement Role"=enum."UUT"}  # Hardware Settings Cluster
              }
              frame Default {
                w185 = T14 {"Sensor ID *"=0, "Target Sample Rate (Hz) *"=0.0, "Steady-State Duration (s) *"=0, "Allowed Tolerance (%) FS *"=0.0, "Max Settling Timeout (s) *"=0, "Physical Channel"="", "Measurement Role"=enum."UUT"}  # Hardware Settings Cluster
              }
            }
            n45 = call "DB Fetch UI List.vi"("Refnum in"=w158, "Identifier"=w148, "UI List Type"=UI_List_Type."Serial Numbers", "UI Device Type"=w146, "Measurement Role"=Measurement_Role_Selection."All", "error in (no error)"=w161) -> ("Refnum out"=w157:T7, "1D Results"=w152:string[], "error out"=w160:errorcluster)  [unwired: 6 in, 1 out]
            n46 = Bundle By Name(cluster=w156, "Serial Numbers"=w152, "Hardware Settings Cluster"=w153) -> (w155:T13)
            n47 = Send Notification(notification=w155, notifier=w147, error in (no error)=w160) -> (error out=w159:errorcluster)  [unwired: 1 out]
          }
          frame "Fetch Calibration Points" {
            w191 = T9 {"1D Notifier"=refnum, "UI List Type"=enum."Model Numbers", "UI Device Type"=enum."Measurement", "Identifier"=0, "2D Notifier"=refnum, "Measurement Role Selection"=enum."Controller"}  # DB Query Request 2D Payload
            n48 = Variant To Data(error in=w206, type=w191, Variant=w199) -> (data=w202:T9, error out=w204:errorcluster)
            n49 = Unbundle By Name(w202) -> ("Identifier"=w190:i32, "2D Notifier"=w198:refnum<notifier>)
            n50 = Number To Decimal String(number=w190) -> (decimal integer string=w189:string)  [unwired: 1 in]
            n51 = Concatenate Strings(w189, "' AND trc.MeasurementRole = 'UUT'\nORDER BY cp.ChannelRecordID, cp.CycleNumber, cp.Setpoint, cp.Direction;") -> (w194:string)
            n52 = Concatenate Strings("SELECT cp.PointID, cp.TestRunID, cp.ChannelRecordID, cp.Setpoint, trc.SensorID, cp.ReferenceValue, cp.MeasuredValue, cp.AccuracyPercentFS, cp.PassFail, cp.Timestamp, cp.CycleNumber, cp.Direction\nFROM CalibrationPoints AS cp\nJOIN TestRuns AS tr ON cp.TestRunID = tr.TestRunID\nJOIN TestRunChannels AS trc ON cp.ChannelRecordID = trc.ChannelRecordID\nJOIN TestRuns AS selectedRun ON tr.CalibrationSessionID = selectedRun.CalibrationSessionID\nWHERE selectedRun.TestRunID ='", w194) -> (w196:string)
            n53 = call "Fetch Calibration Points.vi"("error in (no error)"=w204, "SQL Query"=w196, "Refnum in"=w203) -> ("error out"=w193:errorcluster, "Results"=w188:string[][], "Refnum out"=w192:T7)  [unwired: 6 in]
            n54 = Send Notification(notification=w188, notifier=w198, error in (no error)=w193) -> (error out=w201:errorcluster)  [unwired: 1 out]
          }
          frame "Fetch Sensor Profile" {
            w217 = T16 {"Notifier"=refnum, "Sensor ID"=0}  # Sensor FetchResponse
            n55 = Variant To Data(error in=w228, type=w217, Variant=w213) -> (data=w224:T16, error out=w209:errorcluster)
            n56 = Unbundle By Name(w224) -> ("Sensor ID"=w210:i32, "Notifier"=w223:refnum<notifier>)
            n57 = Format Into String(format string="%d", error in=w209, w210) -> (resulting string=w211:string, error out=w208:errorcluster)  [unwired: 1 in]
            n58 = Concatenate Strings(w211, "';") -> (w221:string)
            n59 = Concatenate Strings("SELECT SensorID, SerialNumber, ModelNumber, Min, Max, Units, OutputSignal FROM Sensors WHERE SensorID = '", w221) -> (w222:string)
            n60 = call "Fetch Sensor Profile.vi"("error in (no error)"=w208, "SQL Query"=w222, "Refnum in"=w225) -> ("error out"=w216:errorcluster, "Sensor CoreData Cluster"=w214:T17, "Refnum out"=w215:T7)  [unwired: 6 in]
            n61 = Send Notification(notification=w214, notifier=w223, error in (no error)=w216) -> (error out=w220:errorcluster)  [unwired: 1 out]
          }
          frame "Fetch Start Run Times" {
            w233 = T9 {"1D Notifier"=refnum, "UI List Type"=enum."Model Numbers", "UI Device Type"=enum."Measurement", "Identifier"=0, "2D Notifier"=refnum, "Measurement Role Selection"=enum."Controller"}  # DB Query Request Payload
            n62 = Variant To Data(error in=w247, type=w233, Variant=w241) -> (data=w245:T9, error out=w239:errorcluster)
            n63 = Unbundle By Name(w245) -> ("UI List Type"=w232:T4, "Identifier"=w231:i32, "2D Notifier"=w244:refnum<notifier>)
            n64 = Format Into String(format string="%d", error in=w239, w231) -> (resulting string=w238:string, error out=w236:errorcluster)  [unwired: 1 in]
            n65 = call "DB Fetch UI List.vi"("Refnum in"=w237, "Identifier"=w238, "UI List Type"=w232, "error in (no error)"=w236) -> ("Refnum out"=w234:T7, "2D Results"=w230:string[][], "error out"=w235:errorcluster)  [unwired: 8 in, 1 out]
            n66 = Send Notification(notification=w230, notifier=w244, error in (no error)=w235) -> (error out=w243:errorcluster)  [unwired: 1 out]
          }
          frame "Start Test Run" {
            w268 = T20 {"Acq Settings"={"Instrument Specifications"=[], "Config Settings"={"Simulated Sensor Injection"=0.0, "Base Device Name"="", "Simulation Mode"=""}}, "Processing Settings"={"Sensor CoreData"=[], "Test Parameters"=[], "Measurement Roles"=[], "Test Sequence Context"={"Direction"=enum."Acsending", "Cycle Number"=0, "Setpoint"=0.0}}, "Session Identifiers"={"SerialNumber"=[], "OperatorName"=""}, "Test Sequence Settings"={"Test Sequence State"={"Test Sequence Enum"=enum."Idle", "Point Index"=0, "Current Target"=0.0, "Previous Target"=0.0, "Simulation?"=FALSE, "Direction"=enum."Acsending", "Transition Active?"=FALSE, "Cycle Number"=0}}, "Stimulus Settings"={"Stimulus Outputs"=[]}}  # Settings
            n67 = Variant To Data(error in=w269, type=w268, Variant=w290) -> (data=w259:T20, error out=w267:errorcluster)
            n68 = Unbundle By Name(w259) -> ("Acq Settings.Instrument Specifications"=w264:T22, "Session Identifiers.OperatorName"=w265:string)
            n69 = Unbundle By Name(w254) -> ("CalibrationSessionID"=w253:i32)
            n70 = Concatenate Strings(w265, "';") -> (w288:string)
            n71 = Get Date/Time In Seconds() -> (seconds since 1Jan1904=w283:timestamp)
            n72 = Concatenate Strings("SELECT OperatorID FROM Operators WHERE OperatorName = '", w288) -> (w286:string)
            n73 = Format Date/Time String(time format string (%c)="%Y-%m-%d %H:%M:%S", seconds (now)=w283) -> (date/time string=w281:string)  [unwired: 1 in]
            n74 = call "Fetch OperatorID.vi"("error in (no error)"=w267, "SQL query"=w286, "Refnum in"=w266) -> ("error out"=w285:errorcluster, "OperatorID"=w280:i32, "Refnum out"=w284:T7)  [unwired: 6 in]
            n75 = for {
              tunnel: w281 -> [w351]
              tunnel: w280 -> [w354]
              tunnel: w264 -> [w350] mode=indexing
              shift-right: [w352] -> w275
              shift-left: w285 -> [w356]
              shift-right: [w353] -> w279
              shift-left: w284 -> [w355]
              tunnel: w253 -> [w348]
              stop <- w349 stop-if-true
              n76 = Unbundle By Name(w350) -> ("Sensor ID *"=w347:i32)
              n77 = Not Equal To 0?(x=w347) -> (x != 0?=w349:bool)
              n78 = case shown="True" w349 {
                tunnel: w356 -> [w357 w366]
                tunnel: w355 -> [w358 w365]
                tunnel: w354 -> [_ w364]
                tunnel: [w358 w363] -> w353
                tunnel: [w357 w362] -> w352
                tunnel: w351 -> [_ w361]
                tunnel: w348 -> [_ w359]
                frame False {
                }
                frame True {
                  w360 = T40 {"RunStartTime"="RunStartTime", "OperatorID"=0, "TestResult"="TestResult", "CalibrationSessionID"=0}  # TestRuns Table Insert
                  n79 = Bundle By Name(cluster=w360, "CalibrationSessionID"=w359, "RunStartTime"=w361, "OperatorID"=w364) -> (w367:T40)
                  n80 = call <vilib>:"DB Tools Insert Data.vi"("data"=w367, "error in (no error)"=w366, "columns"=string[] ["RunStartTime", "OperatorID", "TestResult", "CalibrationSessionID"], "table"="TestRuns", "connection reference"=w365) -> ("error out"=w362:errorcluster, "connection reference out"=w363:T7)  [unwired: 5 in]
                }
              }
            }
            n81 = Unbundle By Name(w259) -> ("Acq Settings.Instrument Specifications"=w258:T22)
            n82 = call-poly <vilib>:"DB Tools Execute Query.vi"("error in (no error)"=w275, "SQL query"="SELECT last_insert_rowid() AS TestRunID;", "connection reference"=w279) -> ("error out"=w276:errorcluster, "recordset reference"=w278:T8)  [unwired: 5 in]
            n83 = Bundle By Name(cluster=w254, "OperatorID"=w280) -> (w270:T6)
            n84 = call-poly <vilib>:"DB Tools Fetch Element Data.vi"("error in (no error)"=w276, "type"=0, "column index"="TestRunID" ("SQL query"), "recordset reference"=w278) -> ("error out"=w274:errorcluster, "data"=w260:i32, "recordset reference out"=w277:T8)  [unwired: 3 in]
            n85 = Bundle By Name(cluster=w270, "TestRunID"=w260) -> (w257:T6)
            n86 = call-poly <vilib>:"DB Tools Free Object.vi"("error in (no error)"=w274, "recordset reference"=w277) -> ("error out"=w261:errorcluster, "connection reference"=w263:T7)  [unwired: 8 in]
            n87 = for {
              tunnel: w260 -> [w306]
              shift-right: [w309] -> w262
              shift-left: w263 -> [w310]
              shift-right: [w307] -> w255
              shift-left: w261 -> [w308]
              tunnel: w258 -> [w305] mode=indexing
              shift-right: [w298] -> w251
              shift-left: i32[] [] -> [w294]
              shift-right: [w295] -> w252
              shift-left: i32[] [] -> [w293]
              i -> [w304]
              n88 = Unbundle By Name(w305) -> ("Sensor ID *"=w296:i32, "Measurement Role"=w297:T5, "Physical Channel"=w302:string)
              n89 = Not Equal To 0?(x=w296) -> (x != 0?=w303:bool)
              n90 = case shown="True" w303 {
                tunnel: w310 -> [w321 w327]
                tunnel: [w321 w331] -> w309
                tunnel: w308 -> [w320 w326]
                tunnel: [w320 w330] -> w307
                tunnel: w306 -> [_ w342]
                tunnel: w296 -> [_ w341]
                tunnel: w304 -> [_ w340]
                tunnel: [0 ("data") w332] -> w299
                tunnel: w297 -> [_ w324]
                tunnel: w302 -> [_ w322]
                frame False {
                }
                frame True {
                  w344 = T41 {"TestRunID"=0, "SensorID"=0, "HardwareRow"=0, "PhysicalChannel"="", "FinalStatus"="", "MeasurementRole"=""}  # DB TestRunChannel Record
                  n91 = call "Get Enum Text.vi"("error in (no error)"=w326, "Enum"=w324) -> ("error out"=w325:errorcluster, "Enum Text"=w323:string)  [unwired: 8 in]
                  n92 = Bundle By Name(cluster=w344, "TestRunID"=w342, "SensorID"=w341, "HardwareRow"=w340, "MeasurementRole"=w323, "PhysicalChannel"=w322) -> (w343:T41)
                  n93 = call <vilib>:"DB Tools Insert Data.vi"("data"=w343, "error in (no error)"=w325, "columns"=string[] ["TestRunID", "SensorID", "HardwareRow", "PhysicalChannel", "FinalStatus", "MeasurementRole"], "table"="TestRunChannels", "connection reference"=w327) -> ("error out"=w329:errorcluster, "connection reference out"=w328:T7)  [unwired: 5 in]
                  n94 = call-poly <vilib>:"DB Tools Execute Query.vi"("error in (no error)"=w329, "SQL query"="SELECT last_insert_rowid() AS ChannelRecordID;", "connection reference"=w328) -> ("error out"=w338:errorcluster, "recordset reference"=w336:T8)  [unwired: 5 in]
                  n95 = call-poly <vilib>:"DB Tools Fetch Element Data.vi"("error in (no error)"=w338, "type"=0, "column index"="ChannelRecordID" ("SQL query"), "recordset reference"=w336) -> ("error out"=w339:errorcluster, "data"=w332:i32, "recordset reference out"=w337:T8)  [unwired: 3 in]
                  n96 = call-poly <vilib>:"DB Tools Free Object.vi"("error in (no error)"=w339, "recordset reference"=w337) -> ("error out"=w330:errorcluster, "connection reference"=w331:T7)  [unwired: 8 in]
                }
              }
              n97 = Equal?(x=w297, y=Measurement_Role."UUT" ("Measurement Role")) -> (x = y?=w300:bool)
              n98 = case shown="False" w300 {
                tunnel: w299 -> [_ w318]
                tunnel: [w312 w317] -> w298
                tunnel: [w311 w315] -> w295
                tunnel: w296 -> [_ w314]
                tunnel: w294 -> [w312 w316]
                tunnel: w293 -> [w311 w313]
                frame False {
                }
                frame True {
                  n99 = Build Array (concatenate)(w316, w318) -> (w317:i32[])
                  n100 = Build Array (concatenate)(w313, w314) -> (w315:i32[])
                }
              }
            }
            n101 = Bundle By Name(cluster=w257, "ChannelRecordIDs"=w251, "SensorID"=w252) -> (w256:T6)
          }
          frame "Insert Sensor Data" {
            w370 = T42 {"SerialNumber"="", "ModelNumber"="", "Min"=0.0, "Max"=0.0, "Units"=enum."PSI", "Output Signal"=enum."4-20mA"}  # Sensor Table Insert
            w395 = T43 {"Notifier"=refnum, "Sensor CoreData"={"SerialNumber"="", "ModelNumber"="", "Min"=0.0, "Max"=0.0, "Units"=enum."PSI", "Output Signal"=enum."4-20mA", "SensorID"=0}}  # Sensor InsertRequest
            n102 = Variant To Data(error in=w399, type=w395, Variant=w398) -> (data=w396:T43, error out=w378:errorcluster)
            n103 = Unbundle By Name(w396) -> ("Sensor CoreData.SerialNumber"=w377:string, "Sensor CoreData.ModelNumber"=w376:string, "Sensor CoreData.Min"=w375:dbl, "Sensor CoreData.Max"=w374:dbl, "Sensor CoreData.Units"=w372:T18, "Sensor CoreData.Output Signal"=w371:T19, "Notifier"=w373:refnum<notifier>)
            n104 = Bundle By Name(cluster=w370, "SerialNumber"=w377, "ModelNumber"=w376, "Min"=w375, "Max"=w374, "Units"=w372, "Output Signal"=w371) -> (w382:T42)
            n105 = call <vilib>:"DB Tools Insert Data.vi"("data"=w382, "error in (no error)"=w378, "columns"=string[] ["SerialNumber", "ModelNumber", "Min", "Max", "Units", "OutputSignal"], "table"="Sensors", "connection reference"=w394) -> ("error out"=w380:errorcluster, "connection reference out"=w379:T7)  [unwired: 5 in]
            n106 = Unbundle By Name(w380) -> ("code"=w391:i32, "source"=w384:string)
            n107 = Build Array("UNIQUE", "NOT NULL", "BUSY") -> (w387:string[])
            n108 = case shown="-2147467259, -2147217900" w391 {
              selector: w391 -> [w403 w412 w420]
              tunnel: w384 -> [w402 _ w425]
              tunnel: w387 -> [_ _ w427]
              tunnel: [w401 w410 w422] -> w385
              tunnel: [w407 w415 w419] -> w383
              frame 0 {
                w405 = T44 {"status"=FALSE, "code"=0, "source"=""}  # Error Cluster
                w408 = T45 {"Error Cluster"={"status"=FALSE, "code"=0, "source"=""}, "Message"=""}  # Error Payload
                n109 = Bundle By Name(cluster=w405, "status"=FALSE, "code"=w403, "source"=w402) -> (w401:T44)
                n110 = Bundle By Name(cluster=w408, "Error Cluster"=w401, "Message"="Entry inserted into Database successfully" ("source")) -> (w407:T45)
              }
              frame Default {
                w409 = "Critical System Error: Database transaction aborted. Contact Engineering"
                w414 = T44 {"status"=FALSE, "code"=0, "source"=""}  # Error Cluster
                w416 = T45 {"Error Cluster"={"status"=FALSE, "code"=0, "source"=""}, "Message"=""}  # Error Payload
                n111 = Bundle By Name(cluster=w414, "status"=TRUE, "code"=w412, "source"=w409) -> (w411:T44)
                n112 = Bundle By Name(cluster=w416, "Error Cluster"=w411, "Message"=w409) -> (w415:T45)
                n113 = call <vilib>:"Clear Errors.vi"("error in (no error)"=w411) -> ("error out"=w410:errorcluster)  [unwired: 5 in, 1 out]
              }
              frame -2147467259, -2147217900 {
                w423 = T45 {"Error Cluster"={"status"=FALSE, "code"=0, "source"=""}, "Message"=""}  # Error Payload
                n114 = To Upper Case(1:w425) -> (0:w424:string)
                n115 = while {
                  tunnel: w424 -> [w440]
                  tunnel: w427 -> [w436] mode=indexing
                  tunnel: [w436] -> w426
                  stop <- w437 stop-if-true
                  n116 = Search/Split String(string=w440, search string/char (-)=w436) -> (offset of match=w439:i32)  [unwired: 1 in, 2 out]
                  n117 = Not Equal?(x=w439, y=-1) -> (x != y?=w437:bool)
                }
                n118 = case shown="\"UNIQUE\"" w426 {
                  tunnel: ["Database Error Occurred" "Serial Number already exists" "Fields cannot be blank" "Database busy, try again"] -> w417
                  tunnel: [TRUE TRUE TRUE TRUE] -> w421
                  frame Default {
                  }
                  frame "UNIQUE" {
                  }
                  frame "NOT NULL" {
                  }
                  frame "busy" {
                  }
                }
                n119 = Bundle By Name(cluster=w423, "Error Cluster.code"=w420, "Error Cluster.status"=w421, "Error Cluster.source"=w417, "Message"=w417) -> (w419:T45)
                n120 = Unbundle By Name(w419) -> ("Error Cluster"=w418:T44)
                n121 = call <vilib>:"Clear Errors.vi"("error in (no error)"=w418) -> ("error out"=w422:errorcluster)  [unwired: 5 in, 1 out]
              }
            }
            n122 = Send Notification(notification=w383, notifier=w373, error in (no error)=w385) -> (error out=w386:errorcluster)  [unwired: 1 out]
          }
          frame "Insert Channel" {
            w442 = T46 {"RunID"=0, "SensorID"=0, "HardwareRow"=0, "PhysicalChannel"=""}  # Channel CoreData Cluster
            w465 = T47 {"Notifier"=refnum, "Channel CoreData"={"RunID"=0, "SensorID"=0, "HardwareRow"=0, "PhysicalChannel"=""}}  # Channel InsertRequest
            n123 = Variant To Data(error in=w468, type=w465, Variant=w467) -> (data=w466:T47, error out=w448:errorcluster)
            n124 = Unbundle By Name(w466) -> ("Channel CoreData.RunID"=w447:i32, "Channel CoreData.SensorID"=w446:i32, "Channel CoreData.HardwareRow"=w445:i32, "Channel CoreData.PhysicalChannel"=w444:string, "Notifier"=w443:refnum<notifier>)
            n125 = Bundle By Name(cluster=w442, "RunID"=w447, "SensorID"=w446, "HardwareRow"=w445, "PhysicalChannel"=w444) -> (w452:T46)
            n126 = call <vilib>:"DB Tools Insert Data.vi"("data"=w452, "error in (no error)"=w448, "columns"=string[] ["RunID", "SensorID", "HardwareRow", "PhysicalChannel"], "table"="TestRunChannels", "connection reference"=w464) -> ("error out"=w450:errorcluster, "connection reference out"=w449:T7)  [unwired: 5 in]
            n127 = Unbundle By Name(w450) -> ("code"=w461:i32, "source"=w454:string)
            n128 = Build Array("UNIQUE", "NOT NULL", "BUSY") -> (w457:string[])
            n129 = case shown="-2147467259, -2147217900" w461 {
              selector: w461 -> [w472 w481 w489]
              tunnel: w454 -> [w471 _ w494]
              tunnel: w457 -> [_ _ w496]
              tunnel: [w470 w479 w491] -> w455
              tunnel: [w476 w484 w488] -> w453
              frame 0 {
                w474 = T44 {"status"=FALSE, "code"=0, "source"=""}  # Error Cluster
                w477 = T45 {"Error Cluster"={"status"=FALSE, "code"=0, "source"=""}, "Message"=""}  # Error Payload
                n130 = Bundle By Name(cluster=w474, "status"=FALSE, "code"=w472, "source"=w471) -> (w470:T44)
                n131 = Bundle By Name(cluster=w477, "Error Cluster"=w470, "Message"="Entry inserted into Database successfully" ("source")) -> (w476:T45)
              }
              frame Default {
                w478 = "Critical System Error: Database transaction aborted. Contact Engineering"
                w483 = T44 {"status"=FALSE, "code"=0, "source"=""}  # Error Cluster
                w485 = T45 {"Error Cluster"={"status"=FALSE, "code"=0, "source"=""}, "Message"=""}  # Error Payload
                n132 = Bundle By Name(cluster=w483, "status"=TRUE, "code"=w481, "source"=w478) -> (w480:T44)
                n133 = Bundle By Name(cluster=w485, "Error Cluster"=w480, "Message"=w478) -> (w484:T45)
                n134 = call <vilib>:"Clear Errors.vi"("error in (no error)"=w480) -> ("error out"=w479:errorcluster)  [unwired: 5 in, 1 out]
              }
              frame -2147467259, -2147217900 {
                w492 = T45 {"Error Cluster"={"status"=FALSE, "code"=0, "source"=""}, "Message"=""}  # Error Payload
                n135 = To Upper Case(1:w494) -> (0:w493:string)
                n136 = while {
                  tunnel: w493 -> [w509]
                  tunnel: w496 -> [w505] mode=indexing
                  tunnel: [w505] -> w495
                  stop <- w506 stop-if-true
                  n137 = Search/Split String(string=w509, search string/char (-)=w505) -> (offset of match=w508:i32)  [unwired: 1 in, 2 out]
                  n138 = Not Equal?(x=w508, y=-1) -> (x != y?=w506:bool)
                }
                n139 = case shown="Default" w495 {
                  tunnel: ["Database Error Occurred" "Serial Number already exists" "Fields cannot be blank" "Database busy, try again"] -> w486
                  tunnel: [TRUE TRUE TRUE TRUE] -> w490
                  frame Default {
                  }
                  frame "UNIQUE" {
                  }
                  frame "NOT NULL" {
                  }
                  frame "busy" {
                  }
                }
                n140 = Bundle By Name(cluster=w492, "Error Cluster.code"=w489, "Error Cluster.status"=w490, "Error Cluster.source"=w486, "Message"=w486) -> (w488:T45)
                n141 = Unbundle By Name(w488) -> ("Error Cluster"=w487:T44)
                n142 = call <vilib>:"Clear Errors.vi"("error in (no error)"=w487) -> ("error out"=w491:errorcluster)  [unwired: 5 in, 1 out]
              }
            }
            n143 = Send Notification(notification=w453, notifier=w443, error in (no error)=w455) -> (error out=w456:errorcluster)  [unwired: 1 out]
          }
          frame "Insert Operator Data" {
            w530 = T48 {"Notifier"=refnum, "OperatorName"="", "BadgeNumber"="", "IsActive"=0}  # Operator Payload
            n144 = Variant To Data(error in=w532, type=w530, Variant=w510) -> (data=w515:T48, error out=w516:errorcluster)
            n145 = Unbundle By Name(w515) -> ("OperatorName"=w514:string, "Notifier"=w525:refnum<notifier>)
            n146 = call <vilib>:"DB Tools Insert Data.vi"("data"=w514, "error in (no error)"=w516, "columns"=string[] ["OperatorName"], "table"="Operators", "connection reference"=w529) -> ("error out"=w512:errorcluster, "connection reference out"=w511:T7)  [unwired: 5 in]
            n147 = Build Array("UNIQUE", "NOT NULL", "BUSY") -> (w521:string[])
            n148 = Unbundle By Name(w512) -> ("code"=w526:i32, "source"=w518:string)
            n149 = case shown="Default" w526 {
              selector: w526 -> [w536 w545 w553]
              tunnel: w518 -> [w535 _ w558]
              tunnel: w521 -> [_ _ w560]
              tunnel: [w534 w543 w555] -> w519
              tunnel: [w540 w548 w552] -> w517
              frame 0 {
                w538 = T44 {"status"=FALSE, "code"=0, "source"=""}  # Error Cluster
                w541 = T45 {"Error Cluster"={"status"=FALSE, "code"=0, "source"=""}, "Message"=""}  # Error Payload
                n150 = Bundle By Name(cluster=w538, "status"=FALSE, "code"=w536, "source"=w535) -> (w534:T44)
                n151 = Bundle By Name(cluster=w541, "Error Cluster"=w534, "Message"="Entry inserted into Database successfully" ("source")) -> (w540:T45)
              }
              frame Default {
                w542 = "Critical System Error: Database transaction aborted. Contact Engineering"
                w547 = T44 {"status"=FALSE, "code"=0, "source"=""}  # Error Cluster
                w549 = T45 {"Error Cluster"={"status"=FALSE, "code"=0, "source"=""}, "Message"=""}  # Error Payload
                n152 = Bundle By Name(cluster=w547, "status"=TRUE, "code"=w545, "source"=w542) -> (w544:T44)
                n153 = Bundle By Name(cluster=w549, "Error Cluster"=w544, "Message"=w542) -> (w548:T45)
                n154 = call <vilib>:"Clear Errors.vi"("error in (no error)"=w544) -> ("error out"=w543:errorcluster)  [unwired: 5 in, 1 out]
              }
              frame -2147467259, -2147217900 {
                w556 = T45 {"Error Cluster"={"status"=FALSE, "code"=0, "source"=""}, "Message"=""}  # Error Payload
                n155 = To Upper Case(1:w558) -> (0:w557:string)
                n156 = while {
                  tunnel: w557 -> [w573]
                  tunnel: w560 -> [w569] mode=indexing
                  tunnel: [w569] -> w559
                  stop <- w570 stop-if-true
                  n157 = Search/Split String(string=w573, search string/char (-)=w569) -> (offset of match=w572:i32)  [unwired: 1 in, 2 out]
                  n158 = Not Equal?(x=w572, y=-1) -> (x != y?=w570:bool)
                }
                n159 = case shown="\"UNIQUE\"" w559 {
                  tunnel: ["Database Error Occurred" "Serial Number already exists" "Fields cannot be blank" "Database busy, try again"] -> w550
                  tunnel: [TRUE TRUE TRUE TRUE] -> w554
                  frame Default {
                  }
                  frame "UNIQUE" {
                  }
                  frame "NOT NULL" {
                  }
                  frame "busy" {
                  }
                }
                n160 = Bundle By Name(cluster=w556, "Error Cluster.code"=w553, "Error Cluster.status"=w554, "Error Cluster.source"=w550, "Message"=w550) -> (w552:T45)
                n161 = Unbundle By Name(w552) -> ("Error Cluster"=w551:T44)
                n162 = call <vilib>:"Clear Errors.vi"("error in (no error)"=w551) -> ("error out"=w555:errorcluster)  [unwired: 5 in, 1 out]
              }
            }
            n163 = Send Notification(notification=w517, notifier=w525, error in (no error)=w519) -> (error out=w520:errorcluster)  [unwired: 1 out]
          }
          frame "Insert Calibration Session" {
            n164 = call-poly <vilib>:"DB Tools Execute Query.vi"("error in (no error)"=w575, "SQL query"="INSERT INTO CalibrationSessions (SessionStartTime)\nVALUES (CURRENT_TIMESTAMP);", "connection reference"=w592) -> ("error out"=w574:errorcluster, "recordset reference"=w589:T8)  [unwired: 5 in]
            n165 = call-poly <vilib>:"DB Tools Free Object.vi"("error in (no error)"=w574, "recordset reference"=w589) -> ("error out"=w587:errorcluster, "connection reference"=w588:T7)  [unwired: 8 in]
            n166 = call-poly <vilib>:"DB Tools Execute Query.vi"("error in (no error)"=w587, "SQL query"="SELECT last_insert_rowid() AS CalibrationSessionID;", "connection reference"=w588) -> ("error out"=w584:errorcluster, "recordset reference"=w583:T8)  [unwired: 5 in]
            n167 = call-poly <vilib>:"DB Tools Fetch Element Data.vi"("error in (no error)"=w584, "type"=0, "column index"="CalibrationSessionID" ("SQL query"), "recordset reference"=w583) -> ("error out"=w581:errorcluster, "data"=w577:i32, "recordset reference out"=w582:T8)  [unwired: 3 in]
            n168 = call-poly <vilib>:"DB Tools Free Object.vi"("error in (no error)"=w581, "recordset reference"=w582) -> ("error out"=w580:errorcluster, "connection reference"=w579:T7)  [unwired: 8 in]
            n169 = Bundle By Name(cluster=w578, "CalibrationSessionID"=w577) -> (w576:T6)
          }
          frame "Insert Calibration Points" {
            w602 = T49 []  # Processed Calibration Points
            n170 = Unbundle By Name(w599) -> ("SensorID"=w595:i32[], "TestRunID"=w596:i32, "ChannelRecordIDs"=w598:i32[])
            n171 = Variant To Data(error in=w614, type=w602, Variant=w597) -> (data=w601:T49, error out=w611:errorcluster)
            n172 = for {
              shift-right: [w632] -> w610
              shift-left: w612 -> [w635]
              shift-right: [w631] -> w604
              shift-left: w611 -> [w630]
              tunnel: w601 -> [w628] mode=indexing
              tunnel: w598 -> [w622] mode=indexing
              tunnel: w596 -> [w621]
              tunnel: w595 -> [w617] mode=indexing
              w629 = T52 {"TestRunID"=0, "ChannelRecordID"=0, "Setpoint"=0.0, "MeasuredValue"=0.0, "AccuracyPercentFS"=0.0, "PassFail"=FALSE, "ReferenceValue"=0.0, "Cycle Number"=0, "Direction"="", "SensorID"=0}  # Calibration Point Table Insert
              n173 = Unbundle By Name(w628) -> ("Setpoint"=w623:dbl, "Measured Value"=w627:dbl, "AccuracyPercentFS"=w616:dbl, "Pass/Fail"=w626:bool, "Reference Value"=w625:dbl, "Cycle Number"=w620:i32, "Direction"=w619:T29)
              n174 = case shown="\"Descending\"" w619 {
                tunnel: ["Acsending" "Error" "Descending"] -> w618
                frame "Acsending" {
                }
                frame Default {
                }
                frame "Descending" {
                }
              }
              n175 = Bundle By Name(cluster=w629, "SensorID"=w617, "TestRunID"=w621, "ChannelRecordID"=w622, "Setpoint"=w623, "MeasuredValue"=w627, "AccuracyPercentFS"=w616, "PassFail"=w626, "ReferenceValue"=w625, "Cycle Number"=w620, "Direction"=w618) -> (w624:T52)
              n176 = call <vilib>:"DB Tools Insert Data.vi"("data"=w624, "error in (no error)"=w630, "columns"=string[] ["TestRunID", "ChannelRecordID", "Setpoint", "MeasuredValue", "AccuracyPercentFS", "PassFail", "ReferenceValue", "CycleNumber", "Direction", "SensorID"], "table"="CalibrationPoints", "connection reference"=w635) -> ("error out"=w631:errorcluster, "connection reference out"=w632:T7)  [unwired: 5 in]
            }
            n177 = Unbundle By Name(w604) -> ("code"=w609:i32, "source"=w603:string)
            n178 = Build Array("UNIQUE", "NOT NULL", "BUSY") -> (w605:string[])
            n179 = case shown="-2147467259, -2147217900" w609 {
              selector: w609 -> [w641 w649 w656]
              tunnel: w603 -> [w640 _ w661]
              tunnel: w605 -> [_ _ w663]
              tunnel: [w639 w647 w658] -> w600
              frame 0 {
                w643 = T44 {"status"=FALSE, "code"=0, "source"=""}  # Error Cluster
                w645 = T45 {"Error Cluster"={"status"=FALSE, "code"=0, "source"=""}, "Message"=""}  # Error Payload
                n180 = Bundle By Name(cluster=w643, "status"=FALSE, "code"=w641, "source"=w640) -> (w639:T44)
                n181 = Bundle By Name(cluster=w645, "Error Cluster"=w639, "Message"="Entry inserted into Database successfully" ("source")) -> ()  [unwired: 1 out]
              }
              frame Default {
                w646 = "Critical System Error: Database transaction aborted. Contact Engineering"
                w651 = T44 {"status"=FALSE, "code"=0, "source"=""}  # Error Cluster
                w652 = T45 {"Error Cluster"={"status"=FALSE, "code"=0, "source"=""}, "Message"=""}  # Error Payload
                n182 = Bundle By Name(cluster=w651, "status"=TRUE, "code"=w649, "source"=w646) -> (w648:T44)
                n183 = Bundle By Name(cluster=w652, "Error Cluster"=w648, "Message"=w646) -> ()  [unwired: 1 out]
                n184 = call <vilib>:"Clear Errors.vi"("error in (no error)"=w648) -> ("error out"=w647:errorcluster)  [unwired: 5 in, 1 out]
              }
              frame -2147467259, -2147217900 {
                w659 = T45 {"Error Cluster"={"status"=FALSE, "code"=0, "source"=""}, "Message"=""}  # Error Payload
                n185 = To Upper Case(1:w661) -> (0:w660:string)
                n186 = while {
                  tunnel: w660 -> [w676]
                  tunnel: w663 -> [w672] mode=indexing
                  tunnel: [w672] -> w662
                  stop <- w673 stop-if-true
                  n187 = Search/Split String(string=w676, search string/char (-)=w672) -> (offset of match=w675:i32)  [unwired: 1 in, 2 out]
                  n188 = Not Equal?(x=w675, y=-1) -> (x != y?=w673:bool)
                }
                n189 = case shown="\"UNIQUE\"" w662 {
                  tunnel: ["Database Error Occurred" "Serial Number already exists" "Fields cannot be blank" "Database busy, try again"] -> w653
                  tunnel: [TRUE TRUE TRUE TRUE] -> w657
                  frame Default {
                  }
                  frame "UNIQUE" {
                  }
                  frame "NOT NULL" {
                  }
                  frame "busy" {
                  }
                }
                n190 = Bundle By Name(cluster=w659, "Error Cluster.code"=w656, "Error Cluster.status"=w657, "Error Cluster.source"=w653, "Message"=w653) -> (w655:T45)
                n191 = Unbundle By Name(w655) -> ("Error Cluster"=w654:T44)
                n192 = call <vilib>:"Clear Errors.vi"("error in (no error)"=w654) -> ("error out"=w658:errorcluster)  [unwired: 5 in, 1 out]
              }
            }
          }
          frame "Log System Error" {
            w680 = T53 {"status"=FALSE, "error_code"=0, "description"="", "source_loop"=""}  # error constant
            n193 = Variant To Data(error in=w695, type=w680, Variant=w694) -> (data=w679:T53, error out=w681:errorcluster)
            n194 = Equal To 0?(x=w689) -> (x = 0?=w693:bool)
            n195 = case shown="True" w693 {
              tunnel: w681 -> [w709 w714]
              tunnel: [w709 w712] -> w687
              tunnel: w688 -> [w708 w711]
              tunnel: [w708 w710] -> w686
              frame False {
              }
              frame True {
                n196 = call-poly <vilib>:"DB Tools Execute Query.vi"("error in (no error)"=w714, "SQL query"="BEGIN TRANSACTION;" ("Message"), "connection reference"=w711) -> ("error out"=w713:errorcluster, "recordset reference"=w716:T8)  [unwired: 5 in]
                n197 = call-poly <vilib>:"DB Tools Free Object.vi"("error in (no error)"=w713, "recordset reference"=w716) -> ("error out"=w712:errorcluster, "connection reference"=w710:T7)  [unwired: 8 in]
              }
            }
            n198 = call "Write System Error To DB.vi"("error in (no error)"=w687, "Error_Payload"=w679, "Refnum in"=w686) -> ("error out"=w683:errorcluster, "Refnum out"=w685:T7)  [unwired: 7 in]
            n199 = Increment(x=w689) -> (x+1=w678:i32)
            n200 = Greater Or Equal?(x=w678, y=10) -> (x >= y?=w691:bool)
            n201 = case shown="True" w691 {
              tunnel: [w699 0] -> w690
              tunnel: w678 -> [w699 _]
              tunnel: w685 -> [w698 w703]
              tunnel: [w698 w702] -> w684
              tunnel: w683 -> [w697 w701]
              tunnel: [w697 w700] -> w682
              frame False {
              }
              frame True {
                n202 = call-poly <vilib>:"DB Tools Execute Query.vi"("error in (no error)"=w701, "SQL query"="COMMIT;" ("Message"), "connection reference"=w703) -> ("error out"=w705:errorcluster, "recordset reference"=w704:T8)  [unwired: 5 in]
                n203 = call-poly <vilib>:"DB Tools Free Object.vi"("error in (no error)"=w705, "recordset reference"=w704) -> ("error out"=w700:errorcluster, "connection reference"=w702:T7)  [unwired: 8 in]
              }
            }
          }
          frame "Exit" {
            n204 = Greater Than 0?(x=w723) -> (x > 0?=w722:bool)
            n205 = case shown="False" w722 {
              tunnel: w717 -> [w727 w732]
              tunnel: [w727 w729] -> w720
              tunnel: w721 -> [w726 w731]
              tunnel: [w726 w730] -> w719
              frame False {
              }
              frame True {
                n206 = call-poly <vilib>:"DB Tools Execute Query.vi"("error in (no error)"=w732, "SQL query"="COMMIT;" ("Message"), "connection reference"=w731) -> ("error out"=w728:errorcluster, "recordset reference"=w734:T8)  [unwired: 5 in]
                n207 = call-poly <vilib>:"DB Tools Free Object.vi"("error in (no error)"=w728, "recordset reference"=w734) -> ("error out"=w729:errorcluster, "connection reference"=w730:T7)  [unwired: 8 in]
              }
            }
            n208 = call <vilib>:"DB Tools Close Connection.vi"("error in (no error)"=w720, "connection reference"=w719) -> ("error out"=w725:errorcluster)  [unwired: 5 in]
          }
          frame Default {
            n209 = xnode "Error Ring"("parameter 0"=w739) -> ("error out"=w738:errorcluster)
          }
        }
        n210 = call "Error Handler - DB Handling Loop.vi"("error in (no error)"=w12, "Message Queue"=w17) -> ("dup error in"=w24:errorcluster)  [unwired: 8 in, 1 out]
      }
    }
    frame Error {
    }
  }
  "error out" <- w3
